vi "MicroVisco1.8.vi"() -> ()   [LabVIEW 2014]
doc: "Uses the picture indicator to display a waterfall plot. This example is similar to the Waterfall Spectrum example, which uses a multiplot graph to display a waterfall plot. However, this example can fill the area under the waveforms, because you can use the Picture VIs to fill shapes. Also, by drawing the data from back to front, this VI does not need to do the hidden line removal that the other example does.\n\nNote: You must have the LabVIEW Full or Professional Development Systems to run this example."
uses:
  Library/Image Acq..vi
  <vilib>/Utility/error.llb/DialogType.ctl
  <vilib>/Instr/_visa.llb/Select Event Type.ctl
  Library/IT_Sent.vi
  Library/SD_Sent.vi
  Library/Sent_Settings.vi
  Library/Set_OK.vi
  Library/Set_Cancel.vi
  Library/Temp_Sent.vi
  Library/Set_File_Name.vi
  Library/malfunc. stop.vi
  <vilib>/Instr/_visa.llb/VISA Configure Serial Port (Instr).vi
  <vilib>/imaqUSB/imaqUSB.llb/IMAQ USB.ctl
  <vilib>/vision/Image Controls.llb/IMAQ Image.ctl
panel:
  in  "Image File Path (jpg)":path
  out "Emer Stop ACK":string
  out "Syringe ACK":string
  out "Capture ACK":string
  out "Injection ACK":string
  out "Mode ACK":string
  out "AutoStart ACK":string
  out "Wash ACK":string
  out "Setting ACK Read":string
  out "Autostart Ind":bool=TRUE
  out "Numeric":i32
  out "Image Out (duplicate)":T1
  in  "Mal Func Stop":bool
  out "IMAQ USB Session Out 2":T2
  out "Settings ACK":bool
  out "IT Sent":dbl
  out "SD sent":dbl
  out "Sent Settings":string
  out "OK":bool
  out "Cancel":bool
  out "Temp Sent":dbl
  out "PBS Viscosity":dbl
  out "PBS Count":dbl
  out "Blood Viscosity":dbl
  out "Blood Count":dbl
  in  "Settings":bool
  out "Setting\nTemp":dbl(slide) caption="Setting \nTemperature" scale=0.0..100.0
  out "Setting \nDischarge":dbl(slide) scale=0.0..1000.0
  out "Current\nTemp":dbl(slide) caption="Current \nTemperature" scale=0.0..100.0
  out "Current \nDischarge":dbl(slide) scale=0.0..1000.0
  out "CT":dbl format="%#.1f"
  in  "Converttype":u8
  out "CD Low":string
  out "CT Low":string
  out "Stop read buffer":string
  out "Stop 2":bool
  out "CD":dbl
  out "Current RX Data":string
  out "EMER STOP ACK":bool
  out "AUTO/STRT ACK":bool
  out "MODE CTR ACK":bool
  out "SYRINGE ACK":bool
  out "CAP ACK":bool
  out "Inj ACK":bool
  out "WashACK":bool
  out "Read RX":refnum<visa-resource-name>
  in  "AutoStart":bool
  out "Syringe Ind":bool
  out "Wash Ind":bool=TRUE
  out "Inj Ind":bool
  out "Cap Ind":bool
  in  "Syringe Back":bool
  in  "capture":bool
  in  "Injection":bool
  in  "Wash":bool
  out "DATAs\nControl":i8(ring)=48 items=["STOP"=48, "Begin"=49]
  out "Commands":i8(ring)=77 items=["Torque"=84, "Fling Dist"=77, "Rotate Left"=67, "Rotate Right"=83, "Stop"=86, "Auto"=69]
  out "Checksum":i8 format="%x"
  in  "Emergency\nStop":bool
  in  "Mode Control":bool
  in  "Select COM Port":refnum<visa-resource-name>="COM1"
  out "Image Acq.":bool
  out "USB Camera Names":string[](array[string])
  out "Image out":T1
  out "IMAQ USB Session Out":T2
  out "USB Camera":string
  out "Image":T1(plugin-control)
  out "COM Port":refnum<visa-resource-name>="COM3"
  # "MICRO VISCO-METER"
  # "Auto Start"
  # "Measurements"
  # "cP"
  # "cP"
  # "o"
  # "C"
  # "uL/h"
  # "o"
  # "C"
  # "uL/h"
  # "=>"
  # "=>"
  # "=>"
  # "Syringe Release"
  # "Capture"
  # "Injection"
  # "Wash"
  # "Manual"
  # "Auto"
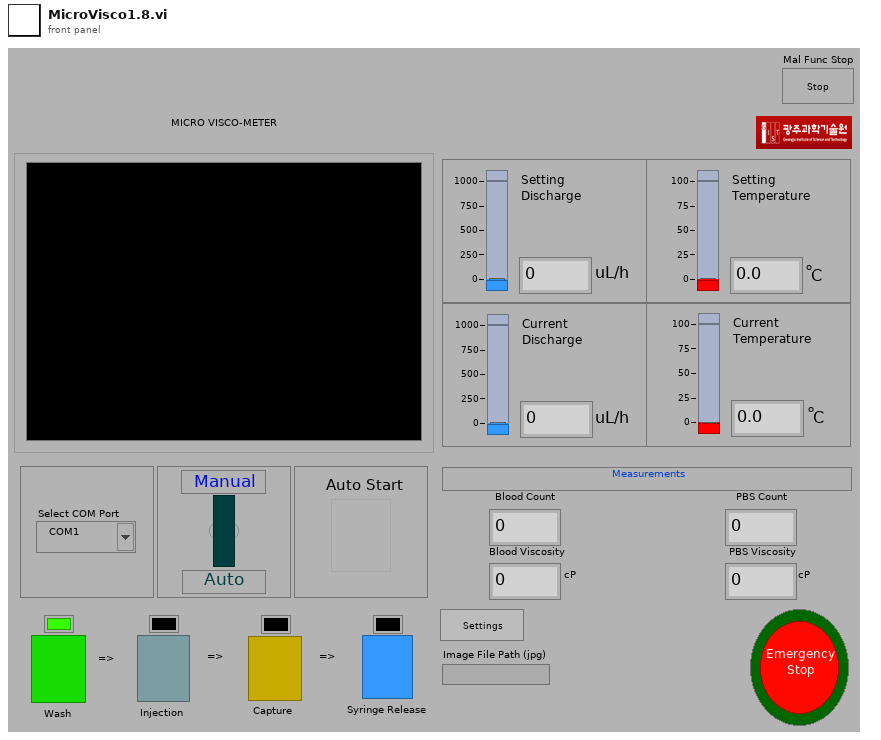
[diagram p1: front panel]
types:
  T1 = typedef "IMAQ Image.ctl" = refnum<image>
  T2 = typedef "IMAQ USB.ctl" = refnum<k1>
  T3 = enum16{"open", "replace", "create", "open or create", "replace or create", "replace or create with confirmation"}
  T4 = cluster{"xmin":dbl, "xmax":dbl, "ymin":dbl, "ymax":dbl}
  T5 = typedef "DialogType.ctl" = u16
  T6 = typedef "Select Event Type.ctl" = u32
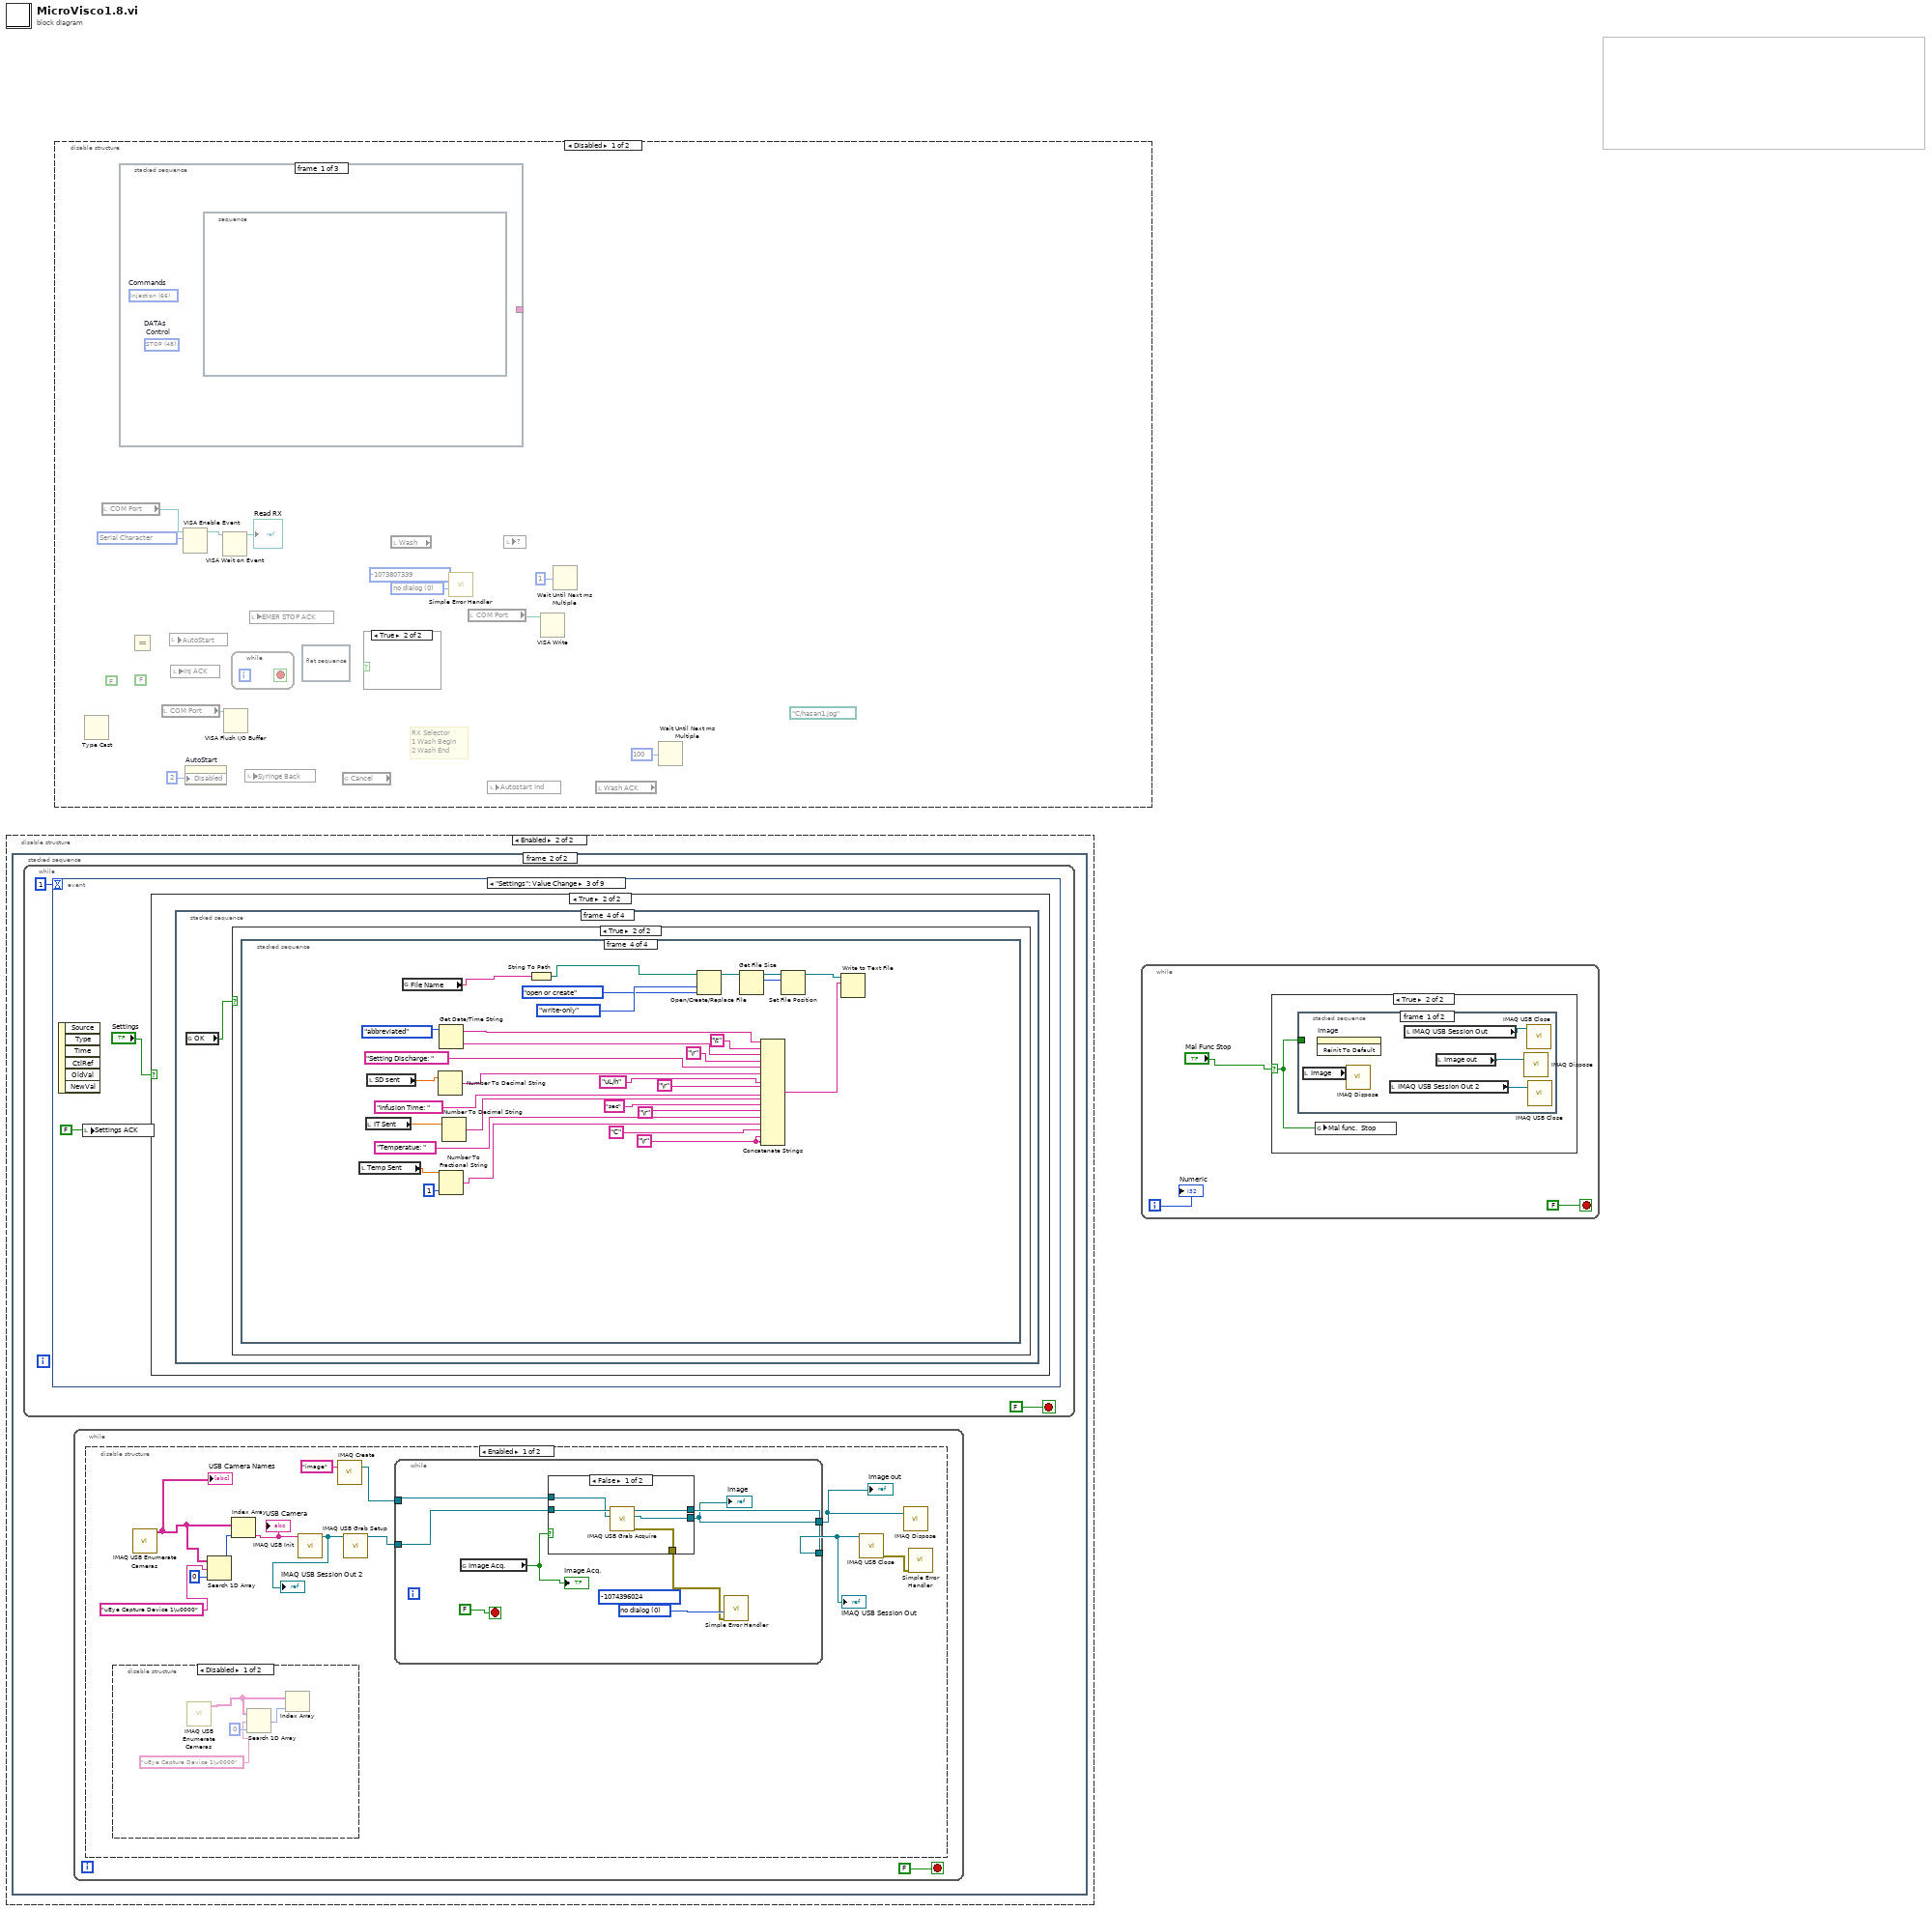
[diagram p0: block diagram]
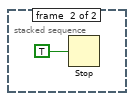
[diagram p3: hidden frame]
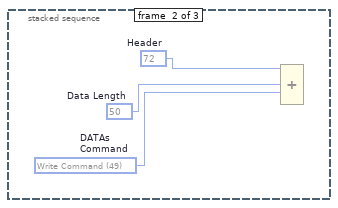
[diagram p5: hidden frame]
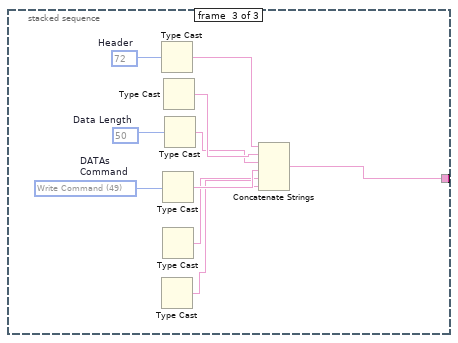
[diagram p6: hidden frame]
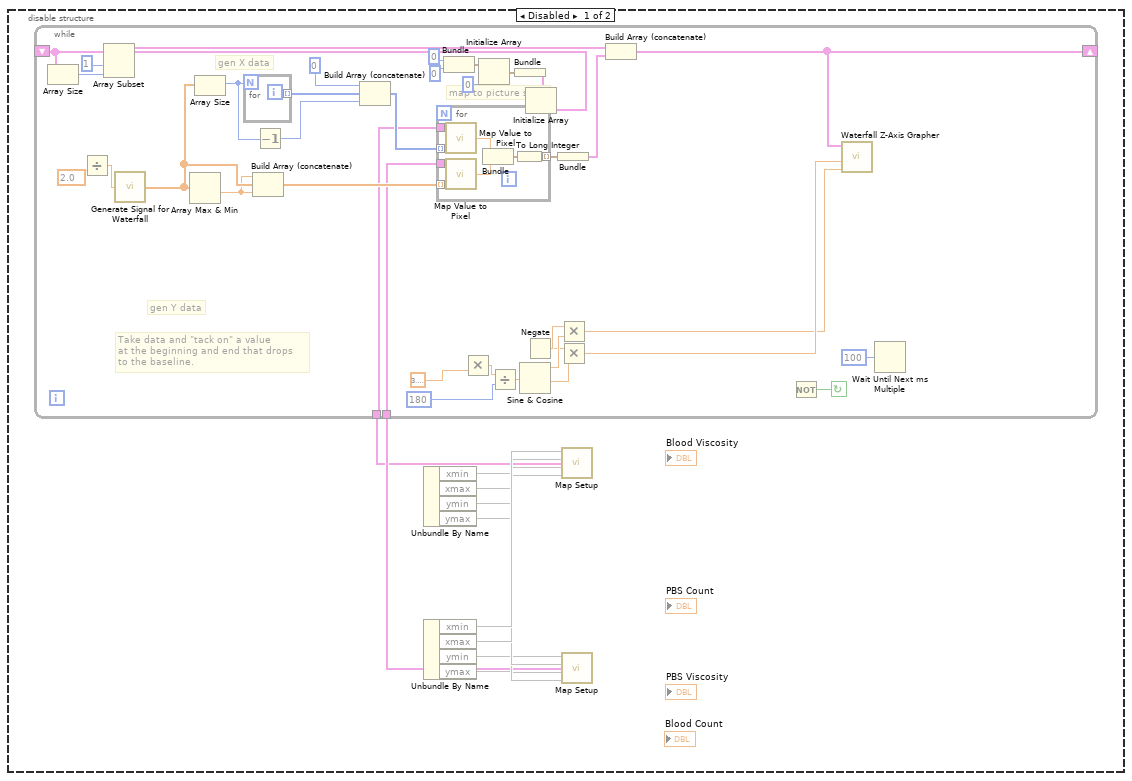
[diagram p8: hidden frame]
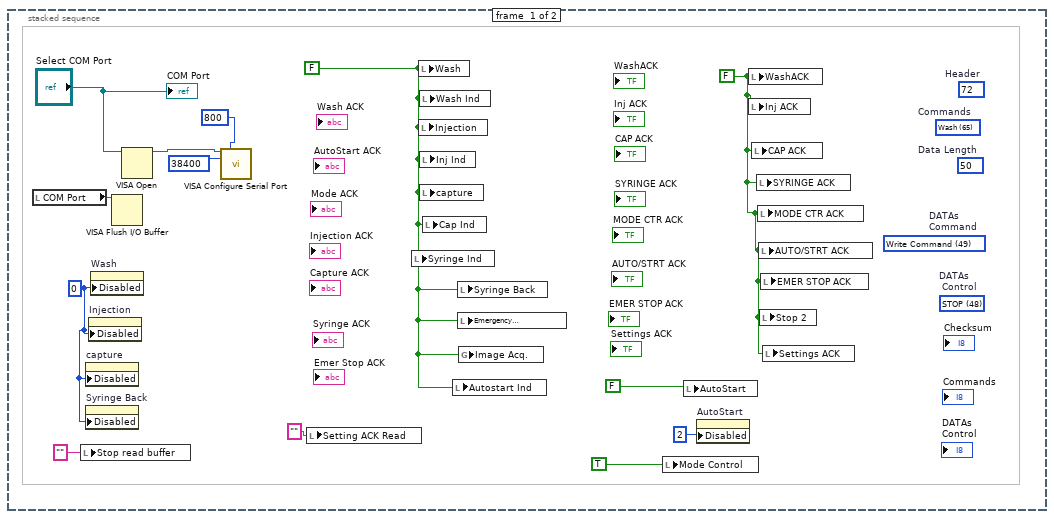
[diagram p9: hidden frame]
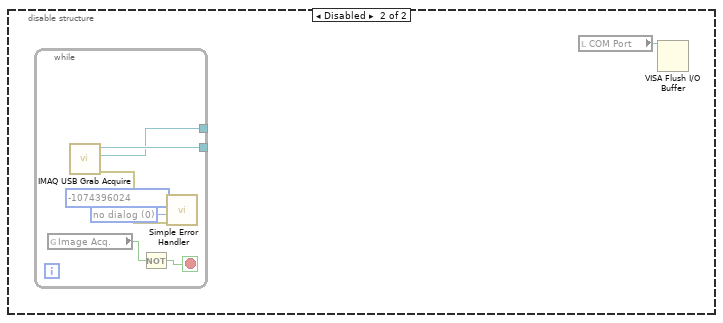
[diagram p12: hidden frame]
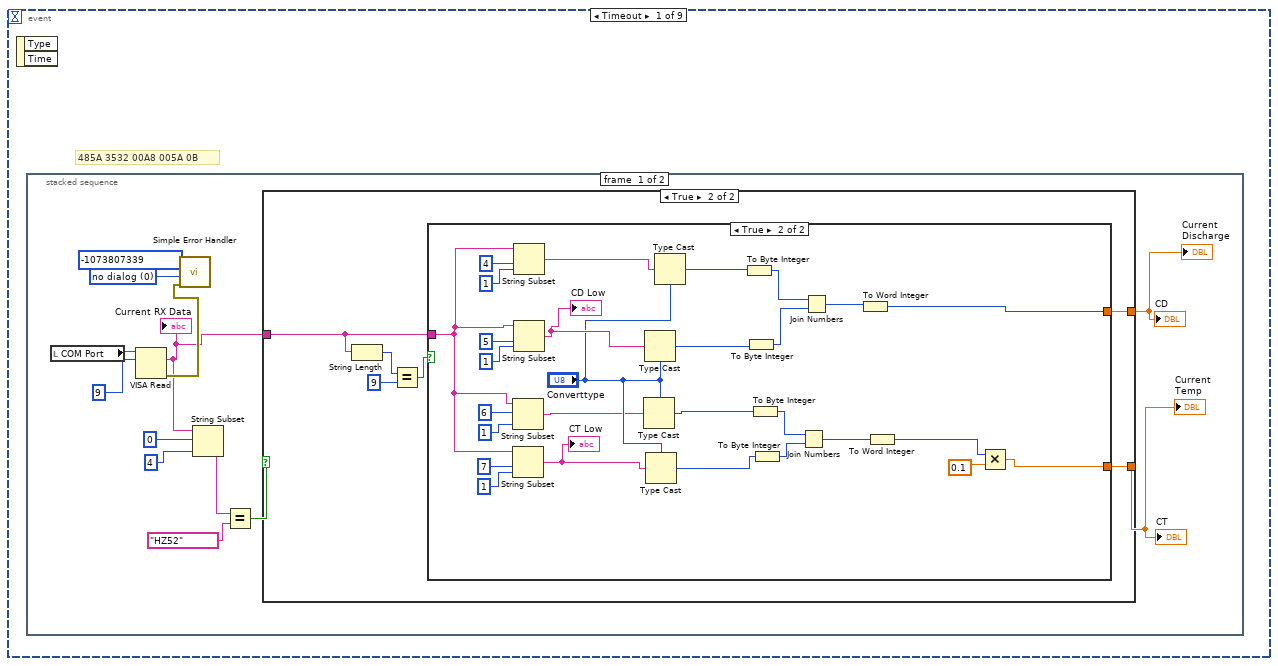
[diagram p13: hidden frame]
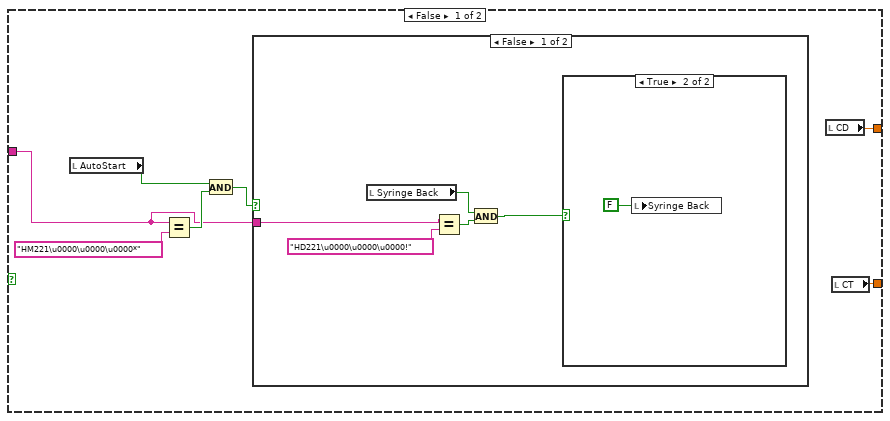
[diagram p14: hidden frame]
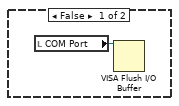
[diagram p15: hidden frame]
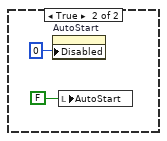
[diagram p16: hidden frame]
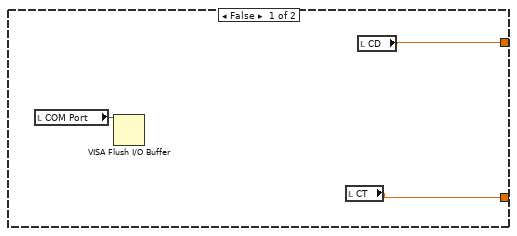
[diagram p17: hidden frame]
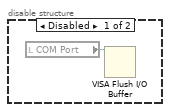
[diagram p19: hidden frame]
diagram:
  n1 = disable-structure shown="Enabled" {
    frame Disabled {
      n2 = Unbundle By Name() -> (w11:cluster{}, "xmin"=w8, "xmax"=w7, "ymin"=w6, "ymax"=w5)
      n3 = Unbundle By Name() -> (w12:T4, "xmin"=w10, "xmax"=w9, "ymin"=w4, "ymax"=w3)
      n4 = Bundle(0, 0) -> (w19:cluster{i32, i32})  [unwired: 1 in]
      n5 = Initialize Array(w19, 0) -> (w15:cluster{i32, i32}[])
      n6 = Bundle(w15) -> (w14:cluster{cluster{i32, i32}[]})  [unwired: 1 in]
      n7 = Initialize Array(w14) -> (w13:cluster{cluster{i32, i32}[]}[])  [unwired: 1 in]
      n8 = call <vilib>:"Map Setup.vi"("coordinate 1"=w10, "value 1"=w8, "coordinate 2"=w9, "value 2"=w7) -> ("scale factors"=w1:cluster{"a":dbl, "b":dbl, "log?(F)":bool})  [unwired: 1 in]
      n9 = call <vilib>:"Map Setup.vi"("coordinate 1"=w4, "value 1"=w6, "coordinate 2"=w3, "value 2"=w5) -> ("scale factors"=w2:cluster{"a":dbl, "b":dbl, "log?(F)":bool})  [unwired: 1 in]
      n10 = while {
        tunnel: w1 -> [w21]
        tunnel: w2 -> [w22]
        shift-left: w13 -> [w50]
        shift-right: [w30] -> _
        stop <- w53 continue-if-true
        # "map to picture size"
        # "Take data and \"tack on\" a value\nat the beginning and end that drops\nto the baseline."
        # "gen Y data"
        # "gen X data"
        n11 = Array Size(array=w50) -> (size(s)=w49:i32)
        n12 = Divide(y=2.0) -> (x/y=w35:dbl)  [unwired: 1 in]
        n13 = Array Subset(array=w50, index=1, length=w49) -> (w43:cluster{cluster{i32, i32}[]}[])
        n14 = call "Generate Signal for Waterfall.vi"("amplitude"=w35) -> ("waveform"=w34:dbl[], "# cycles"=w52:dbl)  [unwired: 1 in]
        n15 = Array Max & Min(array=w34) -> (min value=w33:dbl)  [unwired: 3 out]
        n16 = Array Size(array=w34) -> (size(s)=w44:i32)
        n17 = for {
          N: w44 -> [_]
          tunnel: [w63] -> w47 mode=indexing
          i -> [w63]
        }
        n18 = Build Array (concatenate)(w33, w34, w33) -> (w24:dbl[])
        n19 = Decrement(x=w44) -> (x-1=w45:i32)
        n20 = Build Array (concatenate)(0, w47, w45) -> (w25:i32[])
        n21 = for {
          tunnel: w25 -> [w62] mode=indexing
          tunnel: w24 -> [w61] mode=indexing
          tunnel: [w55] -> w23 mode=indexing
          tunnel: w22 -> [w57]
          tunnel: w21 -> [w56]
          n22 = call <vilib>:"Map Value to Pixel.vi"("x"=w62, "scale factors"=w56) -> ("pixel"=w59:dbl)  [unwired: 1 in]
          n23 = call <vilib>:"Map Value to Pixel.vi"("x"=w61, "scale factors"=w57) -> ("pixel"=w60:dbl)  [unwired: 1 in]
          n24 = Bundle("pixel"=w59, "pixel"=w60) -> (w58:cluster{"pixel":dbl, "pixel":dbl})  [unwired: 1 in]
          n25 = To Long Integer(number=w58) -> (32bit integer=w55:cluster{"pixel":i32, "pixel":i32})
        }
        n26 = Multiply(y=3.141592653589793) -> (x*y=w40:dbl)  [unwired: 1 in]
        n27 = Divide(x=w40, y=180) -> (x/y=w39:dbl)
        n28 = Sine & Cosine(0:w39) -> (1:w27:dbl, 2:w37:dbl)
        n29 = Negate() -> (x=w38:dbl, -x=w26:dbl)
        n30 = Bundle(w23) -> (w48:cluster{cluster{"pixel":i32, "pixel":i32}[]})  [unwired: 1 in]
        n31 = Multiply(x=w38, y=w27) -> (x*y=w31:dbl)
        n32 = Multiply(x=w26, y=w37) -> (x*y=w32:dbl)
        n33 = Build Array (concatenate)(w43, w48) -> (w30:cluster{cluster{"pixel":i32, "pixel":i32}[]}[])
        n34 = Not() -> (x=w54:bool, .not. x?=w53:bool)
        n35 = call "Waterfall Z-Axis Grapher.vi"("horizontal offset between plots"=w31, "vertical offset between plots"=w32, "graph"=w30) -> ("waterfall plot"=w28:picture, "colors"=w29:u32[])
        n36 = Wait Until Next ms Multiple(millisecond multiple=u32 100) -> ()  [unwired: 1 out]
      }
    }
    frame Enabled {
      n37 = stacked-sequence {
        frame #0 {
          (unwired) i8 65 items=["Syringe"=83, "Temp"=84, "Pump"=80, "Walve "=86, "LED "=76, "JIG "=74, "Wash"=65, "Injection"=66, "Capture"=67, "Readout"=68, "AUTO/MANUAL"=85, "AutoStart"=77, "E.STOP"=69, ""=0]  # Commands
          (unwired) i8 50  # Data Length
          (unwired) i8 72  # Header
          (unwired) i8 49 items=["Write Command"=49]  # DATAs Command
          (unwired) i8 48 items=["STOP"=48, "Begin"=49]  # DATAs  Control
          w70 = u8 0 ("Disabled")
          w67 = FALSE ("WashACK")
          w65 = FALSE ("Wash")
          n38 = local read "COM Port"() -> (w68:refnum<visa-resource-name>)
          n39 = local write "Stop read buffer"("" ("read buffer")) -> ()
          n40 = property on="capture" class="Bool (strict)"("Disabled"=w70) -> ()  [unwired: 2 in, 2 out]
          n41 = property on="Syringe Back" class="Bool (strict)"("Disabled"=w70) -> ()  [unwired: 2 in, 2 out]
          n42 = property on="Injection" class="Bool (strict)"("Disabled"=w70) -> ()  [unwired: 2 in, 2 out]
          n43 = property on="Wash" class="Bool (strict)"("Disabled"=w70) -> ()  [unwired: 2 in, 2 out]
          n44 = VISA Flush I/O Buffer(VISA resource name=w68) -> ()  [unwired: 1 in, 3 out]
          n45 = VISA Open(VISA resource name="Select COM Port") -> (VISA resource name=w76:refnum<visa-resource-name>)  [unwired: 1 in, 4 out]
          n46 = call-poly "VISA Configure Serial Port"("VISA resource name"=w76, "timeout (10sec)"=u32 800, "baud rate (9600)"=u32 38400) -> ()  [unwired: 4 in, 9 out]
          n47 = local write "Setting ACK Read"("" ("read buffer")) -> ()
          n48 = local write "Syringe Ind"(w65) -> ()
          n49 = local write "Wash"(w65) -> ()
          n50 = local write "Injection"(w65) -> ()
          n51 = local write "Wash Ind"(w65) -> ()
          n52 = local write "Inj Ind"(w65) -> ()
          n53 = local write "capture"(w65) -> ()
          n54 = local write "Cap Ind"(w65) -> ()
          n55 = local write "Autostart Ind"(w65) -> ()
          n56 = local write "Syringe Back"(w65) -> ()
          n57 = local write "Emergency\nStop"(w65) -> ()
          n58 = global write "Image Acq..vi" "Image Acq."(w65) -> ()
          n59 = local write "Mode Control"(TRUE ("Image Acq.")) -> ()
          n60 = local write "AutoStart"(FALSE ("AutoStart")) -> ()
          n61 = property on="AutoStart" class="Bool (strict)"("Disabled"=u8 2) -> ()  [unwired: 2 in, 2 out]
          n62 = local write "WashACK"(w67) -> ()
          n63 = local write "Inj ACK"(w67) -> ()
          n64 = local write "CAP ACK"(w67) -> ()
          n65 = local write "SYRINGE ACK"(w67) -> ()
          n66 = local write "MODE CTR ACK"(w67) -> ()
          n67 = local write "AUTO/STRT ACK"(w67) -> ()
          n68 = local write "Stop 2"(w67) -> ()
          n69 = local write "EMER STOP ACK"(w67) -> ()
          n70 = local write "Settings ACK"(w67) -> ()
          "COM Port" <- "Select COM Port"
        }
        frame #1 {
          n71 = while {
            stop <- FALSE stop-if-true
            n72 = event shown="[2] \"Settings\": Value Change" {
              selector: _ -> [_ _ _ _ _ _ _ _ _]
              dyn-events: _ -> [_ _ _ _ _ _ _ _ _]
              timeout: 1 -> [_ _ _ _ _ _ _ _ _]
              event Timeout {
                # "485A 3532 00A8 005A 0B"
                n73 = event-data() -> ()  [unwired: 3 out]
                n74 = stacked-sequence {
                  frame #0 {
                    w131 = T5 0 items=["no dialog", "OK message", "continue or stop message", "OK message + warnings", "continue/stop + warnings"] ("type of dialog (OK msg:1)")
                    n75 = local read "COM Port"() -> (w128:refnum<visa-resource-name>)
                    n76 = VISA Read(VISA resource name=w128, byte count=u32 9) -> (read buffer=w121:string, error out=w130:errorcluster)  [unwired: 1 in, 2 out]
                    "Current RX Data" <- w121
                    n77 = call <vilib>:"Simple Error Handler.vi"("error code (no error:0)"=-1073807339, "type of dialog (OK msg:1)"=w131, "error in (no error)"=w130) -> ()  [unwired: 7 out]
                    n78 = String Subset(string=w121, offset (0)=0, length (rest)=4 ("length (rest)")) -> (substring=w124:string)
                    n79 = Equal?(x=w124, y="HZ52" ("Current RX Data")) -> (x = y?=w122:bool)
                    n80 = case shown="True" w122 {
                      tunnel: w121 -> [w132 w150]
                      tunnel: [w138 w153] -> w120
                      tunnel: [w137 w152] -> w119
                      frame False {
                        n81 = local read "AutoStart"() -> (w135:bool)
                        n82 = Equal?(x=w132, y="HM221\u0000\u0000\u0000*" ("Current RX Data")) -> (x = y?=w134:bool)
                        n83 = And(x=w135, y=w134) -> (x .and. y?=w133:bool)
                        n84 = case shown="False" w133 {
                          tunnel: w132 -> [w141 _]
                          frame False {
                            n85 = local read "Syringe Back"() -> (w140:bool)
                            n86 = Equal?(x=w141, y="HD221\u0000\u0000\u0000!" ("Current RX Data")) -> (x = y?=w143:bool)
                            n87 = And(x=w140, y=w143) -> (x .and. y?=w139:bool)
                            n88 = case shown="True" w139 {
                              frame False {
                                n89 = local read "COM Port"() -> (w144:refnum<visa-resource-name>)
                                n90 = VISA Flush I/O Buffer(VISA resource name=w144) -> ()  [unwired: 1 in, 3 out]
                              }
                              frame True {
                                n91 = local write "Syringe Back"(FALSE ("Syringe Back")) -> ()
                              }
                            }
                          }
                          frame True {
                            n92 = property on="AutoStart" class="Bool (strict)"("Disabled"=u8 0) -> ()  [unwired: 2 in, 2 out]
                            n93 = local write "AutoStart"(FALSE ("AutoStart")) -> ()
                          }
                        }
                        n94 = local read "CD"() -> (w138:dbl)
                        n95 = local read "CT"() -> (w137:dbl)
                      }
                      frame True {
                        n96 = String Length(string=w150) -> (length=w149:i32)
                        n97 = Equal?(x=w149, y=9) -> (x = y?=w151:bool)
                        n98 = case shown="True" w151 {
                          tunnel: w150 -> [_ w175]
                          tunnel: [w156 w158] -> w153
                          tunnel: [w155 w157] -> w152
                          frame False {
                            n99 = local read "COM Port"() -> (w154:refnum<visa-resource-name>)
                            n100 = VISA Flush I/O Buffer(VISA resource name=w154) -> ()  [unwired: 1 in, 3 out]
                            n101 = local read "CT"() -> (w155:dbl)
                            n102 = local read "CD"() -> (w156:dbl)
                          }
                          frame True {
                            n103 = String Subset(string=w175, offset (0)=6, length (rest)=1 ("length (rest)")) -> (substring=w164:string)
                            n104 = String Subset(string=w175, offset (0)=7, length (rest)=1 ("length (rest)")) -> (substring=w161:string)
                            "CT Low" <- w161
                            n105 = String Subset(string=w175, offset (0)=4, length (rest)=1 ("length (rest)")) -> (substring=w167:string)
                            n106 = String Subset(string=w175, offset (0)=5, length (rest)=1 ("length (rest)")) -> (substring=w166:string)
                            "CD Low" <- w166
                            n107 = Type Cast(type="Converttype", x=w164) -> (*(type *) &x=w163:u8)
                            n108 = Type Cast(type="Converttype", x=w166) -> (*(type *) &x=w168:u8)
                            n109 = Type Cast(type="Converttype", x=w161) -> (*(type *) &x=w162:u8)
                            n110 = Type Cast(type="Converttype", x=w167) -> (*(type *) &x=w169:u8)
                            n111 = To Byte Integer(number=w169) -> (8bit integer=w171:i8)
                            n112 = To Byte Integer(number=w168) -> (8bit integer=w170:i8)
                            n113 = To Byte Integer(number=w163) -> (8bit integer=w174:i8)
                            n114 = To Byte Integer(number=w162) -> (8bit integer=w160:i8)
                            n115 = Join Numbers(hi=w174, lo=w160) -> ((hi.lo)=w159:u16)
                            n116 = Join Numbers(hi=w171, lo=w170) -> ((hi.lo)=w176:u16)
                            n117 = To Word Integer(number=w176) -> (16bit integer=w158:i16)
                            n118 = To Word Integer(number=w159) -> (16bit integer=w172:i16)
                            n119 = Multiply(x=w172, y=0.1 ("Numeric")) -> (x*y=w157:dbl)
                          }
                        }
                      }
                    }
                    "CD" <- w120
                    "CT" <- w119
                    "Current \nDischarge" <- w120
                    "Current\nTemp" <- w119
                  }
                  frame #1 {
                    n120 = disable-structure shown="Enabled" {
                      frame Enabled {
                        # "Only for Test"
                      }
                      frame Disabled {
                      }
                    }
                    n121 = disable-structure shown="Enabled" {
                      frame Disabled {
                        n122 = local read "COM Port"() -> (w185:refnum<visa-resource-name>)
                        n123 = VISA Flush I/O Buffer(VISA resource name=w185) -> ()  [unwired: 1 in, 3 out]
                      }
                      frame Enabled {
                      }
                    }
                  }
                }
              }
              event "Mode Control": Value Change {
                w187 = i8 85 items=["Syringe"=83, "Temp"=84, "Pump"=80, "Walve "=86, "LED "=76, "JIG "=74, "Wash"=65, "Injection"=66, "Capture"=67, "Readout"=68, "AUTO/MANUAL"=85, "E.STOP"=69]  # Commands
                n124 = event-data() -> ()  [unwired: 7 out]
                n125 = local write "Commands"(w187) -> ()
                n126 = local write "MODE CTR ACK"(FALSE ("MODE CTR ACK")) -> ()
                n127 = case shown="True" "Mode Control" {
                  frame False {
                    w189 = FALSE ("Wash")
                    n128 = local write "Wash Ind"(w189) -> ()
                    n129 = local write "Injection"(w189) -> ()
                    n130 = local write "Wash"(w189) -> ()
                    n131 = local write "Inj Ind"(w189) -> ()
                    n132 = local write "capture"(w189) -> ()
                    n133 = local write "Cap Ind"(w189) -> ()
                    n134 = local write "Syringe Back"(w189) -> ()
                    n135 = local write "Syringe Ind"(w189) -> ()
                    n136 = stacked-sequence {
                      frame #0 {
                        n137 = local read "COM Port"() -> (w190:refnum<visa-resource-name>)
                        n138 = VISA Flush I/O Buffer(VISA resource name=w190) -> ()  [unwired: 1 in, 3 out]
                      }
                      frame #1 {
                        w191 = i8 49 items=["MANUAL"=50, "AUTO"=49]  # DATAs  Control
                        n139 = local write "DATAs\nControl"(w191) -> ()
                      }
                      frame #2 {
                        w194 = i8 49 items=["Write Command"=49]  # DATAs Command
                        w196 = i8 50  # Data Length
                        w197 = i8 72  # Header
                        n140 = local read "Commands"() -> (w195:i8)
                        n141 = local read "DATAs\nControl"() -> (w193:i8)
                        n142 = Compound Arithmetic op=ADD(w197, w195, w196, w194, w193) -> (w192:i8)
                        n143 = local write "Checksum"(w192) -> ()
                      }
                      frame #3 {
                        n144 = flat-sequence {
                          frame #0 {
                            w210 = i8 50  # Data Length
                            w211 = i8 72  # Header
                            w209 = i8 49 items=["Write Command"=49]  # DATAs Command
                            n145 = local read "DATAs\nControl"() -> (w201:i8)
                            n146 = local read "Checksum"() -> (w200:i8)
                            n147 = local read "Commands"() -> (w202:i8)
                            n148 = Type Cast(x=w211) -> (*(type *) &x=w208:string)  [unwired: 1 out]
                            n149 = Type Cast(x=w200) -> (*(type *) &x=w203:string)  [unwired: 1 out]
                            n150 = Type Cast(x=w209) -> (*(type *) &x=w205:string)  [unwired: 1 out]
                            n151 = Type Cast(x=w201) -> (*(type *) &x=w204:string)  [unwired: 1 out]
                            n152 = Type Cast(x=w202) -> (*(type *) &x=w207:string)  [unwired: 1 out]
                            n153 = Type Cast(x=w210) -> (*(type *) &x=w206:string)  [unwired: 1 out]
                            n154 = Concatenate Strings(w208, w207, w206, w205, w204, w203) -> (w198:string)
                            n155 = local read "COM Port"() -> (w199:refnum<visa-resource-name>)
                            n156 = VISA Write(VISA resource name=w199, write buffer=w198) -> ()  [unwired: 1 in, 3 out]
                          }
                          frame #1 {
                            n157 = local read "COM Port"() -> (w212:refnum<visa-resource-name>)
                            n158 = VISA Read(VISA resource name=w212, byte count=u32 6) -> (read buffer=w214:string)  [unwired: 1 in, 3 out]
                            n159 = local write "Mode ACK"(w214) -> ()
                          }
                        }
                      }
                      frame #4 {
                        n160 = while {
                          stop <- w215 stop-if-true
                          n161 = flat-sequence {
                            frame #0 {
                              w220 = "HU\u0015\u0000\u0000²"  # Auto Ctrl NACK
                              w218 = "HU2111"  # Auto Control
                              n162 = local read "Mode ACK"() -> (w217:string)
                              n163 = local read "COM Port"() -> (w216:refnum<visa-resource-name>)
                              n164 = Equal?(x=w217, y=w218) -> (x = y?=w221:bool)
                              n165 = Equal?(x=w217, y=w220) -> (x = y?=w219:bool)
                              n166 = case shown="True" w221 {
                                tunnel: w219 -> [w224 _]
                                tunnel: w216 -> [w223 _]
                                tunnel: w218 -> [w222 _]
                                frame False {
                                n167 = case shown="True" w224 {
                                tunnel: w223 -> [w226 w229]
                                tunnel: w222 -> [w225 w228]
                                frame False {
                                n168 = local write "MODE CTR ACK"(FALSE ("MODE CTR ACK")) -> ()
                                n169 = VISA Write(VISA resource name=w226, write buffer=w225) -> ()  [unwired: 1 in, 3 out]
                                }
                                frame True {
                                n170 = local write "MODE CTR ACK"(FALSE ("MODE CTR ACK")) -> ()
                                n171 = VISA Write(VISA resource name=w229, write buffer=w228) -> ()  [unwired: 1 in, 3 out]
                                }
                                }
                                }
                                frame True {
                                w232 = u8 2 ("Disabled")
                                n172 = property on="Injection" class="Bool (strict)"("Disabled"=w232) -> ()  [unwired: 2 in, 2 out]
                                n173 = property on="Wash" class="Bool (strict)"("Disabled"=w232) -> ()  [unwired: 2 in, 2 out]
                                n174 = local write "MODE CTR ACK"(TRUE ("MODE CTR ACK")) -> ()
                                n175 = property on="capture" class="Bool (strict)"("Disabled"=w232) -> ()  [unwired: 2 in, 2 out]
                                n176 = property on="Syringe Back" class="Bool (strict)"("Disabled"=w232) -> ()  [unwired: 2 in, 2 out]
                                n177 = property on="AutoStart" class="Bool (strict)"("Disabled"=u8 0) -> ()  [unwired: 2 in, 2 out]
                                }
                              }
                            }
                            frame #1 {
                              n178 = local read "COM Port"() -> (w234:refnum<visa-resource-name>)
                              n179 = VISA Flush I/O Buffer(VISA resource name=w234) -> ()  [unwired: 1 in, 3 out]
                            }
                          }
                          n180 = local read "MODE CTR ACK"() -> (w215:bool)
                        }
                      }
                    }
                  }
                  frame True {
                    n181 = stacked-sequence {
                      frame #0 {
                        n182 = local read "COM Port"() -> (w235:refnum<visa-resource-name>)
                        n183 = VISA Flush I/O Buffer(VISA resource name=w235) -> ()  [unwired: 1 in, 3 out]
                      }
                      frame #1 {
                        w236 = i8 50 items=["MANUAL"=50, "AUTO"=49]  # DATAs  Control
                        n184 = local write "DATAs\nControl"(w236) -> ()
                      }
                      frame #2 {
                        w239 = i8 49 items=["Write Command"=49]  # DATAs Command
                        w241 = i8 50  # Data Length
                        w242 = i8 72  # Header
                        n185 = local read "DATAs\nControl"() -> (w238:i8)
                        n186 = local read "Commands"() -> (w240:i8)
                        n187 = Compound Arithmetic op=ADD(w242, w240, w241, w239, w238) -> (w237:i8)
                        n188 = local write "Checksum"(w237) -> ()
                      }
                      frame #3 {
                        n189 = flat-sequence {
                          frame #0 {
                            w255 = i8 50  # Data Length
                            w256 = i8 72  # Header
                            w254 = i8 49 items=["Write Command"=49]  # DATAs Command
                            n190 = local read "DATAs\nControl"() -> (w246:i8)
                            n191 = local read "Commands"() -> (w247:i8)
                            n192 = local read "Checksum"() -> (w245:i8)
                            n193 = Type Cast(x=w256) -> (*(type *) &x=w253:string)  [unwired: 1 out]
                            n194 = Type Cast(x=w245) -> (*(type *) &x=w248:string)  [unwired: 1 out]
                            n195 = Type Cast(x=w254) -> (*(type *) &x=w250:string)  [unwired: 1 out]
                            n196 = Type Cast(x=w246) -> (*(type *) &x=w249:string)  [unwired: 1 out]
                            n197 = Type Cast(x=w247) -> (*(type *) &x=w252:string)  [unwired: 1 out]
                            n198 = Type Cast(x=w255) -> (*(type *) &x=w251:string)  [unwired: 1 out]
                            n199 = Concatenate Strings(w253, w252, w251, w250, w249, w248) -> (w243:string)
                            n200 = local read "COM Port"() -> (w244:refnum<visa-resource-name>)
                            n201 = VISA Write(VISA resource name=w244, write buffer=w243) -> ()  [unwired: 1 in, 3 out]
                          }
                          frame #1 {
                            n202 = local read "COM Port"() -> (w259:refnum<visa-resource-name>)
                            n203 = VISA Read(VISA resource name=w259, byte count=u32 6) -> (read buffer=w257:string)  [unwired: 1 in, 3 out]
                            n204 = local write "Mode ACK"(w257) -> ()
                          }
                        }
                      }
                      frame #4 {
                        n205 = while {
                          stop <- w260 stop-if-true
                          n206 = flat-sequence {
                            frame #0 {
                              w261 = "HU2122"  # Manual Ctrl
                              w265 = "HU\u0015\u0000\u0000²"  # Auto Ctrl NACK
                              n207 = local read "Mode ACK"() -> (w263:string)
                              n208 = local read "COM Port"() -> (w262:refnum<visa-resource-name>)
                              n209 = Equal?(x=w263, y=w261) -> (x = y?=w266:bool)
                              n210 = Equal?(x=w263, y=w265) -> (x = y?=w264:bool)
                              n211 = case shown="True" w266 {
                                tunnel: w264 -> [w269 _]
                                tunnel: w262 -> [w268 _]
                                tunnel: w261 -> [w267 _]
                                frame False {
                                n212 = case shown="True" w269 {
                                tunnel: w268 -> [w271 w274]
                                tunnel: w267 -> [w270 w273]
                                frame False {
                                n213 = local write "MODE CTR ACK"(FALSE ("MODE CTR ACK")) -> ()
                                n214 = VISA Write(VISA resource name=w271, write buffer=w270) -> ()  [unwired: 1 in, 3 out]
                                }
                                frame True {
                                n215 = local write "MODE CTR ACK"(FALSE ("MODE CTR ACK")) -> ()
                                n216 = VISA Write(VISA resource name=w274, write buffer=w273) -> ()  [unwired: 1 in, 3 out]
                                }
                                }
                                }
                                frame True {
                                w277 = u8 0 ("Disabled")
                                n217 = property on="Injection" class="Bool (strict)"("Disabled"=w277) -> ()  [unwired: 2 in, 2 out]
                                n218 = property on="Wash" class="Bool (strict)"("Disabled"=w277) -> ()  [unwired: 2 in, 2 out]
                                n219 = local write "MODE CTR ACK"(TRUE ("MODE CTR ACK")) -> ()
                                n220 = property on="capture" class="Bool (strict)"("Disabled"=w277) -> ()  [unwired: 2 in, 2 out]
                                n221 = property on="Syringe Back" class="Bool (strict)"("Disabled"=w277) -> ()  [unwired: 2 in, 2 out]
                                n222 = property on="AutoStart" class="Bool (strict)"("Disabled"=u8 2) -> ()  [unwired: 2 in, 2 out]
                                }
                              }
                            }
                            frame #1 {
                              n223 = local read "COM Port"() -> (w279:refnum<visa-resource-name>)
                              n224 = VISA Flush I/O Buffer(VISA resource name=w279) -> ()  [unwired: 1 in, 3 out]
                            }
                          }
                          n225 = local read "MODE CTR ACK"() -> (w260:bool)
                        }
                      }
                    }
                  }
                }
              }
              event "Settings": Value Change {
                n226 = event-data() -> ()  [unwired: 7 out]
                n227 = local write "Settings ACK"(FALSE ("Settings ACK")) -> ()
                n228 = case shown="True" "Settings" {
                  frame False {
                  }
                  frame True {
                    n229 = stacked-sequence {
                      frame #0 {
                        n230 = local read "COM Port"() -> (w282:refnum<visa-resource-name>)
                        n231 = VISA Flush I/O Buffer(VISA resource name=w282) -> ()  [unwired: 1 in, 3 out]
                      }
                      frame #1 {
                        n232 = call "Settings1.1.vi"() -> ()  [unwired: 1 out]
                      }
                      frame #2 {
                        n233 = global read "Sent_Settings.vi" "Sent Settings"() -> (→"Sent Settings":string)
                        n234 = global read "Temp_Sent.vi" "Temp Sent"() -> (→"Temp Sent" →"Setting\nTemp":dbl)
                        n235 = global read "IT_Sent.vi" "IT Sent"() -> (→"IT Sent":dbl)
                        n236 = global read "SD_Sent.vi" "SD sent"() -> (→"SD sent" →"Setting \nDischarge":dbl)
                        n237 = global read "Set_Cancel.vi" "Cancel"() -> (→"Cancel":bool)
                        n238 = global read "Set_OK.vi" "OK"() -> (→"OK":bool)
                      }
                      frame #3 {
                        n239 = global read "Set_OK.vi" "OK"() -> (w289:bool)
                        n240 = case shown="True" w289 {
                          frame False {
                          }
                          frame True {
                            n241 = stacked-sequence {
                              frame #0 {
                                n242 = local read "COM Port"() -> (w291:refnum<visa-resource-name>)
                                n243 = VISA Flush I/O Buffer(VISA resource name=w291) -> ()  [unwired: 1 in, 3 out]
                                n244 = Wait Until Next ms Multiple(millisecond multiple=u32 1) -> ()  [unwired: 1 out]
                              }
                              frame #1 {
                                n245 = flat-sequence {
                                tunnel: [w298] -> w293
                                tunnel: [w301] -> w294
                                frame #0 {
                                n246 = global read "Sent_Settings.vi" "Sent Settings"() -> (w296:string)
                                n247 = local read "COM Port"() -> (w295:refnum<visa-resource-name>)
                                n248 = VISA Write(VISA resource name=w295, write buffer=w296) -> ()  [unwired: 1 in, 3 out]
                                }
                                frame #1 {
                                n249 = Wait Until Next ms Multiple(millisecond multiple=u32 1) -> ()  [unwired: 1 out]
                                }
                                frame #2 {
                                n250 = local read "COM Port"() -> (w299:refnum<visa-resource-name>)
                                n251 = VISA Read(VISA resource name=w299, byte count=u32 8) -> (read buffer=w298:string)  [unwired: 1 in, 3 out]
                                }
                                frame #3 {
                                n252 = local read "COM Port"() -> (w303:refnum<visa-resource-name>)
                                n253 = VISA Read(VISA resource name=w303, byte count=u32 3) -> (read buffer=w301:string)  [unwired: 1 in, 3 out]
                                }
                                }
                                n254 = Concatenate Strings(w293, w294) -> (→"Setting ACK Read":string)
                              }
                              frame #2 {
                                (unwired) 20
                                n255 = while {
                                stop <- w304 stop-if-true
                                n256 = flat-sequence {
                                frame #0 {
                                w309 = "HY\u0015\u0000\u0000\u0000\u0000\u0000\u0000\u0000¶"  # Auto Ctrl NACK
                                n257 = local read "Setting ACK Read"() -> (w305:string)
                                n258 = local read "Sent Settings"() -> (w306:string)
                                n259 = Equal?(x=w305, y=w306) -> (x = y?=w308:bool)
                                n260 = Equal?(x=w305, y=w309) -> (x = y?=w307:bool)
                                n261 = case shown="False" w308 {
                                tunnel: w307 -> [w311 _]
                                tunnel: w306 -> [w310 _]
                                frame False {
                                n262 = case shown="False" w311 {
                                tunnel: w310 -> [w312 w317]
                                frame False {
                                n263 = stacked-sequence {
                                tunnel: w312 -> [_ w315]
                                frame #0 {
                                n264 = local read "COM Port"() -> (w313:refnum<visa-resource-name>)
                                n265 = VISA Flush I/O Buffer(VISA resource name=w313) -> ()  [unwired: 1 in, 3 out]
                                }
                                frame #1 {
                                n266 = local read "COM Port"() -> (w316:refnum<visa-resource-name>)
                                n267 = local write "Settings ACK"(FALSE ("Settings ACK")) -> ()
                                n268 = VISA Write(VISA resource name=w316, write buffer=w315) -> ()  [unwired: 1 in, 3 out]
                                }
                                }
                                }
                                frame True {
                                n269 = stacked-sequence {
                                tunnel: w317 -> [_ w320]
                                frame #0 {
                                n270 = local read "COM Port"() -> (w318:refnum<visa-resource-name>)
                                n271 = VISA Flush I/O Buffer(VISA resource name=w318) -> ()  [unwired: 1 in, 3 out]
                                }
                                frame #1 {
                                n272 = local read "COM Port"() -> (w321:refnum<visa-resource-name>)
                                n273 = local write "Settings ACK"(FALSE ("Settings ACK")) -> ()
                                n274 = VISA Write(VISA resource name=w321, write buffer=w320) -> ()  [unwired: 1 in, 3 out]
                                }
                                }
                                }
                                }
                                }
                                frame True {
                                n275 = local write "Settings ACK"(TRUE ("Settings ACK")) -> ()
                                }
                                }
                                }
                                }
                                n276 = local read "Settings ACK"() -> (w304:bool)
                                }
                              }
                              frame #3 {
                                w327 = "\r"
                                n277 = local read "Temp Sent"() -> (w325:dbl)
                                n278 = local read "IT Sent"() -> (w342:dbl)
                                n279 = local read "SD sent"() -> (w347:dbl)
                                n280 = global read "Set_File_Name.vi" "File Name"() -> (w323:string)
                                n281 = Number To Decimal String(number=w347) -> (decimal integer string=w346:string)  [unwired: 1 out]
                                n282 = Get Date/Time String(date format (0)=enum16{"short", "long", "abbreviated"}."abbreviated") -> (date string=w351:string, time string=w350:string)  [unwired: 2 out]
                                n283 = Number To Fractional String(number=w325, precision (6)=i16 1) -> (F-format string=w324:string)  [unwired: 2 out]
                                n284 = Number To Decimal String(number=w342) -> (decimal integer string=w341:string)  [unwired: 1 out]
                                n285 = String To Path(string=w323) -> (path=w333:path)
                                n286 = Open/Create/Replace File(file path (use dialog)=w333, operation (0:open)=T3."open or create", access (0:read/write)=enum16{"read/write", "read-only", "write-only"}."write-only") -> (refnum out=w332:refnum<file>)  [unwired: 1 in, 4 out]
                                n287 = Get File Size(file=w332) -> (refnum out=w335:refnum<file>, size (in bytes)=w336:i64)  [unwired: 1 in, 1 out]
                                n288 = Concatenate Strings(w351, "\t", w350, "\r", "Setting Discharge: ", w346, "uL/h" ("string"), "\r", "Infusion Time: ", w341, "sec" ("string"), "\r", "Temperatue: ", w324, "C" ("string"), w327, w327) -> (w331:string)
                                n289 = Set File Position(offset (in bytes) (0)=w336, refnum=w335) -> (refnum out=w334:refnum<file>)  [unwired: 1 in, 2 out]
                                n290 = Write to Text File(file (use dialog)=w334, text=w331) -> ()  [unwired: 1 in, 4 out]
                              }
                            }
                          }
                        }
                      }
                    }
                  }
                }
              }
              event "AutoStart": Value Change {
                w354 = i8 77 items=["Syringe"=83, "Temp"=84, "Pump"=80, "Walve "=86, "LED "=76, "JIG "=74, "Wash"=65, "Injection"=66, "Capture"=67, "Readout"=68, "AUTO/MANUAL"=85, "AutoStart"=77, "E.STOP"=69]  # Commands
                n291 = event-data() -> ()  [unwired: 7 out]
                n292 = local write "Commands"(w354) -> ()
                n293 = local write "AUTO/STRT ACK"(FALSE ("AUTO/STRT ACK")) -> ()
                n294 = disable-structure shown="Enabled" {
                  disable-tunnel: "AutoStart" -> [w356 _]
                  frame Enabled {
                    n295 = case shown="True" w356 {
                      selector: w356 -> [w357 w405]
                      frame False {
                        n296 = local write "Autostart Ind"(w357) -> ()
                        n297 = disable-structure shown="Disabled" {
                          frame Disabled {
                            n298 = stacked-sequence {
                              frame #0 {
                                n299 = local read "COM Port"() -> (w358:refnum<visa-resource-name>)
                                n300 = VISA Flush I/O Buffer(VISA resource name=w358) -> ()  [unwired: 1 in, 3 out]
                              }
                              frame #1 {
                                w359 = i8 48 items=["MANUAL"=48, "AUTO"=49]  # DATAs  Control
                                n301 = local write "DATAs\nControl"(w359) -> ()
                              }
                              frame #2 {
                                w362 = i8 49 items=["Write Command"=49]  # DATAs Command
                                w361 = i8 50  # Data Length
                                w360 = i8 72  # Header
                                n302 = local read "Commands"() -> (w363:i8)
                                n303 = local read "DATAs\nControl"() -> (w364:i8)
                                n304 = Compound Arithmetic op=ADD(w360, w363, w361, w362, w364) -> (w365:i8)
                                n305 = local write "Checksum"(w365) -> ()
                              }
                              frame #3 {
                                w378 = i8 50  # Data Length
                                w379 = i8 72  # Header
                                w377 = i8 49 items=["Write Command"=49]  # DATAs Command
                                n306 = local read "Commands"() -> (w368:i8)
                                n307 = local read "DATAs\nControl"() -> (w367:i8)
                                n308 = local read "Checksum"() -> (w366:i8)
                                n309 = Type Cast(x=w379) -> (*(type *) &x=w376:string)  [unwired: 1 out]
                                n310 = Type Cast(x=w366) -> (*(type *) &x=w371:string)  [unwired: 1 out]
                                n311 = Type Cast(x=w377) -> (*(type *) &x=w373:string)  [unwired: 1 out]
                                n312 = Type Cast(x=w367) -> (*(type *) &x=w372:string)  [unwired: 1 out]
                                n313 = Type Cast(x=w368) -> (*(type *) &x=w375:string)  [unwired: 1 out]
                                n314 = Type Cast(x=w378) -> (*(type *) &x=w374:string)  [unwired: 1 out]
                                n315 = Concatenate Strings(w376, w375, w374, w373, w372, w371) -> (w369:string)
                                n316 = local read "COM Port"() -> (w370:refnum<visa-resource-name>)
                                n317 = VISA Write(VISA resource name=w370, write buffer=w369) -> ()  [unwired: 1 in, 3 out]
                              }
                              frame #4 {
                                n318 = while {
                                stop <- w382 stop-if-true
                                n319 = flat-sequence {
                                tunnel: [w385] -> w383
                                tunnel: [w385] -> w381
                                tunnel: [w384] -> w380
                                tunnel: w383 -> [w393]
                                tunnel: w381 -> [w390]
                                tunnel: w380 -> [w388]
                                frame #0 {
                                n320 = local read "COM Port"() -> (w384:refnum<visa-resource-name>)
                                n321 = VISA Read(VISA resource name=w384, byte count=u32 6) -> (read buffer=w385:string)  [unwired: 1 in, 3 out]
                                }
                                frame #1 {
                                w387 = "HM210("  # AutoStop
                                w391 = "HM\u0015\u0000\u0000ª"  # AutoStart NACK
                                n322 = Equal?(x=w393, y=w387) -> (x = y?=w392:bool)
                                n323 = Equal?(x=w390, y=w391) -> (x = y?=w389:bool)
                                n324 = case shown="False" w392 {
                                tunnel: w389 -> [w396 _]
                                tunnel: w388 -> [w395 _]
                                tunnel: w387 -> [w394 _]
                                frame False {
                                n325 = case shown="False" w396 {
                                tunnel: w395 -> [w398 w401]
                                tunnel: w394 -> [w397 w400]
                                frame False {
                                n326 = local write "AUTO/STRT ACK"(FALSE ("AUTO/STRT ACK")) -> ()
                                n327 = VISA Write(VISA resource name=w398, write buffer=w397) -> ()  [unwired: 1 in, 3 out]
                                }
                                frame True {
                                n328 = local write "AUTO/STRT ACK"(FALSE ("AUTO/STRT ACK")) -> ()
                                n329 = VISA Write(VISA resource name=w401, write buffer=w400) -> ()  [unwired: 1 in, 3 out]
                                }
                                }
                                }
                                frame True {
                                n330 = local write "AUTO/STRT ACK"(TRUE ("AUTO/STRT ACK")) -> ()
                                }
                                }
                                }
                                frame #2 {
                                n331 = local read "COM Port"() -> (w404:refnum<visa-resource-name>)
                                n332 = VISA Flush I/O Buffer(VISA resource name=w404) -> ()  [unwired: 1 in, 3 out]
                                }
                                }
                                n333 = local read "AUTO/STRT ACK"() -> (w382:bool)
                                }
                              }
                            }
                          }
                          frame Enabled {
                          }
                        }
                      }
                      frame True {
                        n334 = stacked-sequence {
                          frame #0 {
                            n335 = local read "COM Port"() -> (w406:refnum<visa-resource-name>)
                            n336 = VISA Flush I/O Buffer(VISA resource name=w406) -> ()  [unwired: 1 in, 3 out]
                          }
                          frame #1 {
                            w407 = i8 49 items=["MANUAL"=48, "AUTO"=49]  # DATAs  Control
                            n337 = local write "DATAs\nControl"(w407) -> ()
                          }
                          frame #2 {
                            w411 = i8 49 items=["Write Command"=49]  # DATAs Command
                            w412 = i8 50  # Data Length
                            w413 = i8 72  # Header
                            n338 = local read "Commands"() -> (w410:i8)
                            n339 = local read "DATAs\nControl"() -> (w409:i8)
                            n340 = Compound Arithmetic op=ADD(w413, w410, w412, w411, w409) -> (w408:i8)
                            n341 = local write "Checksum"(w408) -> ()
                          }
                          frame #3 {
                            n342 = flat-sequence {
                              frame #0 {
                                w427 = i8 50  # Data Length
                                w419 = i8 72  # Header
                                w426 = i8 49 items=["Write Command"=49]  # DATAs Command
                                n343 = local read "Commands"() -> (w418:i8)
                                n344 = local read "DATAs\nControl"() -> (w416:i8)
                                n345 = local read "Checksum"() -> (w417:i8)
                                n346 = Type Cast(x=w419) -> (*(type *) &x=w425:string)  [unwired: 1 out]
                                n347 = Type Cast(x=w417) -> (*(type *) &x=w420:string)  [unwired: 1 out]
                                n348 = Type Cast(x=w426) -> (*(type *) &x=w422:string)  [unwired: 1 out]
                                n349 = Type Cast(x=w416) -> (*(type *) &x=w421:string)  [unwired: 1 out]
                                n350 = Type Cast(x=w418) -> (*(type *) &x=w424:string)  [unwired: 1 out]
                                n351 = Type Cast(x=w427) -> (*(type *) &x=w423:string)  [unwired: 1 out]
                                n352 = Concatenate Strings(w425, w424, w423, w422, w421, w420) -> (w414:string)
                                n353 = local read "COM Port"() -> (w415:refnum<visa-resource-name>)
                                n354 = VISA Write(VISA resource name=w415, write buffer=w414) -> ()  [unwired: 1 in, 3 out]
                              }
                              frame #1 {
                                n355 = local read "COM Port"() -> (w429:refnum<visa-resource-name>)
                                n356 = VISA Read(VISA resource name=w429, byte count=u32 6) -> (read buffer=w428:string)  [unwired: 1 in, 3 out]
                                n357 = local write "AutoStart ACK"(w428) -> ()
                              }
                            }
                          }
                          frame #4 {
                            n358 = while {
                              stop <- w431 stop-if-true
                              n359 = flat-sequence {
                                frame #0 {
                                w433 = "HM\u0015\u0000\u0000ª"  # AutoStart NACK
                                w434 = "HM211)"  # AutoStart
                                n360 = local read "AutoStart ACK"() -> (w432:string)
                                n361 = local read "COM Port"() -> (w435:refnum<visa-resource-name>)
                                n362 = Equal?(x=w432, y=w434) -> (x = y?=w437:bool)
                                n363 = Equal?(x=w432, y=w433) -> (x = y?=w436:bool)
                                n364 = case shown="True" w437 {
                                tunnel: w436 -> [w440 _]
                                tunnel: w435 -> [w439 _]
                                tunnel: w434 -> [w438 _]
                                frame False {
                                n365 = case shown="False" w440 {
                                tunnel: w439 -> [w442 w445]
                                tunnel: w438 -> [w441 w444]
                                frame False {
                                n366 = local write "WashACK"(FALSE ("WashACK")) -> ()
                                n367 = VISA Write(VISA resource name=w442, write buffer=w441) -> ()  [unwired: 1 in, 3 out]
                                }
                                frame True {
                                n368 = local write "WashACK"(FALSE ("WashACK")) -> ()
                                n369 = VISA Write(VISA resource name=w445, write buffer=w444) -> ()  [unwired: 1 in, 3 out]
                                }
                                }
                                }
                                frame True {
                                n370 = local write "WashACK"(TRUE ("WashACK")) -> ()
                                }
                                }
                                }
                                frame #1 {
                                n371 = local read "COM Port"() -> (w448:refnum<visa-resource-name>)
                                n372 = VISA Flush I/O Buffer(VISA resource name=w448) -> ()  [unwired: 1 in, 3 out]
                                }
                              }
                              n373 = local read "AUTO/STRT ACK"() -> (w431:bool)
                            }
                          }
                        }
                        "Autostart Ind" <- w405
                      }
                    }
                  }
                  frame Disabled {
                  }
                }
              }
              event "Wash": Value Change {
                w450 = i8 65 items=["Syringe"=83, "Temp"=84, "Pump"=80, "Walve "=86, "LED "=76, "JIG "=74, "Wash"=65, "Injection"=66, "Capture"=67, "Readout"=68]  # Commands
                n374 = event-data() -> ()  [unwired: 7 out]
                n375 = local write "WashACK"(FALSE ("WashACK")) -> ()
                n376 = local write "Commands"(w450) -> ()
                n377 = case shown="False" "Wash" {
                  selector: "Wash" -> [w452 w500]
                  frame False {
                    n378 = local write "Wash Ind"(w452) -> ()
                    n379 = stacked-sequence {
                      tunnel: [_ _ _ w462 _] -> _
                      frame #0 {
                        n380 = local read "COM Port"() -> (w453:refnum<visa-resource-name>)
                        n381 = VISA Flush I/O Buffer(VISA resource name=w453) -> ()  [unwired: 1 in, 3 out]
                      }
                      frame #1 {
                        w454 = i8 48 items=["STOP"=48, "Begin"=49]  # DATAs  Control
                        n382 = local write "DATAs\nControl"(w454) -> ()
                      }
                      frame #2 {
                        w457 = i8 49 items=["Write Command"=49]  # DATAs Command
                        w458 = i8 50  # Data Length
                        w460 = i8 72  # Header
                        n383 = local read "DATAs\nControl"() -> (w455:i8)
                        n384 = local read "Commands"() -> (w459:i8)
                        n385 = Compound Arithmetic op=ADD(w460, w459, w458, w457, w455) -> (w456:i8)
                        n386 = local write "Checksum"(w456) -> ()
                      }
                      frame #3 {
                        n387 = flat-sequence {
                          tunnel: [w463] -> w461
                          tunnel: [w480] -> w462
                          tunnel: w461 -> [w480]
                          frame #0 {
                            w475 = i8 50  # Data Length
                            w476 = i8 72  # Header
                            w474 = i8 49 items=["Write Command"=49]  # DATAs Command
                            n388 = local read "DATAs\nControl"() -> (w472:i8)
                            n389 = local read "Commands"() -> (w473:i8)
                            n390 = local read "Checksum"() -> (w471:i8)
                            n391 = Type Cast(x=w476) -> (*(type *) &x=w470:string)  [unwired: 1 out]
                            n392 = Type Cast(x=w471) -> (*(type *) &x=w465:string)  [unwired: 1 out]
                            n393 = Type Cast(x=w474) -> (*(type *) &x=w467:string)  [unwired: 1 out]
                            n394 = Type Cast(x=w472) -> (*(type *) &x=w466:string)  [unwired: 1 out]
                            n395 = Type Cast(x=w473) -> (*(type *) &x=w469:string)  [unwired: 1 out]
                            n396 = Type Cast(x=w475) -> (*(type *) &x=w468:string)  [unwired: 1 out]
                            n397 = Concatenate Strings(w470, w469, w468, w467, w466, w465) -> (w463:string)
                            n398 = local read "COM Port"() -> (w464:refnum<visa-resource-name>)
                            n399 = VISA Write(VISA resource name=w464, write buffer=w463) -> ()  [unwired: 1 in, 3 out]
                          }
                          frame #1 {
                            n400 = local read "COM Port"() -> (w478:refnum<visa-resource-name>)
                            n401 = VISA Read(VISA resource name=w478, byte count=u32 6) -> (read buffer=w477:string)  [unwired: 1 in, 3 out]
                            n402 = local write "Wash ACK"(w477) -> ()
                          }
                        }
                      }
                      frame #4 {
                        n403 = while {
                          stop <- w481 stop-if-true
                          n404 = flat-sequence {
                            frame #0 {
                              w486 = "HA\u0015\u0000\u0000ž"  # NACK
                              w484 = "HA210\u001c"  # Wash End
                              n405 = local read "Wash ACK"() -> (w483:string)
                              n406 = local read "COM Port"() -> (w482:refnum<visa-resource-name>)
                              n407 = Equal?(x=w483, y=w484) -> (x = y?=w487:bool)
                              n408 = Equal?(x=w483, y=w486) -> (x = y?=w485:bool)
                              n409 = case shown="True" w487 {
                                tunnel: w485 -> [w490 _]
                                tunnel: w482 -> [w489 _]
                                tunnel: w484 -> [w488 _]
                                frame False {
                                n410 = case shown="False" w490 {
                                tunnel: w489 -> [w492 w495]
                                tunnel: w488 -> [w491 w494]
                                frame False {
                                n411 = local write "WashACK"(FALSE ("WashACK")) -> ()
                                n412 = VISA Write(VISA resource name=w492, write buffer=w491) -> ()  [unwired: 1 in, 3 out]
                                }
                                frame True {
                                n413 = local write "WashACK"(FALSE ("WashACK")) -> ()
                                n414 = VISA Write(VISA resource name=w495, write buffer=w494) -> ()  [unwired: 1 in, 3 out]
                                }
                                }
                                }
                                frame True {
                                n415 = local write "WashACK"(TRUE ("WashACK")) -> ()
                                }
                              }
                            }
                            frame #1 {
                              n416 = local read "COM Port"() -> (w498:refnum<visa-resource-name>)
                              n417 = VISA Flush I/O Buffer(VISA resource name=w498) -> ()  [unwired: 1 in, 3 out]
                            }
                          }
                          n418 = local read "WashACK"() -> (w481:bool)
                        }
                      }
                    }
                  }
                  frame True {
                    w499 = FALSE ("Injection")
                    n419 = local write "Syringe Back"(w499) -> ()
                    n420 = local write "Syringe Ind"(w499) -> ()
                    n421 = local write "Injection"(w499) -> ()
                    n422 = local write "capture"(w499) -> ()
                    n423 = local write "Inj Ind"(w499) -> ()
                    n424 = local write "Cap Ind"(w499) -> ()
                    n425 = stacked-sequence {
                      frame #0 {
                        n426 = local read "COM Port"() -> (w501:refnum<visa-resource-name>)
                        n427 = VISA Flush I/O Buffer(VISA resource name=w501) -> ()  [unwired: 1 in, 3 out]
                      }
                      frame #1 {
                        w502 = i8 49 items=["STOP"=48, "Begin"=49]  # DATAs  Control
                        n428 = local write "DATAs\nControl"(w502) -> ()
                      }
                      frame #2 {
                        w506 = i8 49 items=["Write Command"=49]  # DATAs Command
                        w507 = i8 50  # Data Length
                        w508 = i8 72  # Header
                        n429 = local read "Commands"() -> (w505:i8)
                        n430 = local read "DATAs\nControl"() -> (w504:i8)
                        n431 = Compound Arithmetic op=ADD(w508, w505, w507, w506, w504) -> (w503:i8)
                        n432 = local write "Checksum"(w503) -> ()
                      }
                      frame #3 {
                        n433 = flat-sequence {
                          frame #0 {
                            w521 = i8 50  # Data Length
                            w522 = i8 72  # Header
                            w520 = i8 49 items=["Write Command"=49]  # DATAs Command
                            n434 = local read "DATAs\nControl"() -> (w512:i8)
                            n435 = local read "Commands"() -> (w511:i8)
                            n436 = local read "Checksum"() -> (w513:i8)
                            n437 = Type Cast(x=w522) -> (*(type *) &x=w519:string)  [unwired: 1 out]
                            n438 = Type Cast(x=w511) -> (*(type *) &x=w518:string)  [unwired: 1 out]
                            n439 = Type Cast(x=w513) -> (*(type *) &x=w514:string)  [unwired: 1 out]
                            n440 = Type Cast(x=w520) -> (*(type *) &x=w516:string)  [unwired: 1 out]
                            n441 = Type Cast(x=w512) -> (*(type *) &x=w515:string)  [unwired: 1 out]
                            n442 = Type Cast(x=w521) -> (*(type *) &x=w517:string)  [unwired: 1 out]
                            n443 = Concatenate Strings(w519, w518, w517, w516, w515, w514) -> (w509:string)
                            n444 = local read "COM Port"() -> (w510:refnum<visa-resource-name>)
                            n445 = VISA Write(VISA resource name=w510, write buffer=w509) -> ()  [unwired: 1 in, 3 out]
                          }
                          frame #1 {
                            n446 = local read "COM Port"() -> (w524:refnum<visa-resource-name>)
                            n447 = VISA Read(VISA resource name=w524, byte count=u32 6) -> (read buffer=w523:string)  [unwired: 1 in, 3 out]
                            n448 = local write "Wash ACK"(w523) -> ()
                          }
                        }
                      }
                      frame #4 {
                        n449 = while {
                          stop <- w526 stop-if-true
                          n450 = flat-sequence {
                            frame #0 {
                              w531 = "HA\u0015\u0000\u0000ž"  # NACK
                              w529 = "HA211\u001d"  # Wash Begin
                              n451 = local read "Wash ACK"() -> (w528:string)
                              n452 = local read "COM Port"() -> (w527:refnum<visa-resource-name>)
                              n453 = Equal?(x=w528, y=w529) -> (x = y?=w532:bool)
                              n454 = Equal?(x=w528, y=w531) -> (x = y?=w530:bool)
                              n455 = case shown="True" w532 {
                                tunnel: w530 -> [w535 _]
                                tunnel: w527 -> [w534 _]
                                tunnel: w529 -> [w533 _]
                                frame False {
                                n456 = case shown="False" w535 {
                                tunnel: w534 -> [w537 w540]
                                tunnel: w533 -> [w536 w539]
                                frame False {
                                n457 = local write "WashACK"(FALSE ("WashACK")) -> ()
                                n458 = VISA Write(VISA resource name=w537, write buffer=w536) -> ()  [unwired: 1 in, 3 out]
                                }
                                frame True {
                                n459 = local write "WashACK"(FALSE ("WashACK")) -> ()
                                n460 = VISA Write(VISA resource name=w540, write buffer=w539) -> ()  [unwired: 1 in, 3 out]
                                }
                                }
                                }
                                frame True {
                                n461 = local write "WashACK"(TRUE ("WashACK")) -> ()
                                }
                              }
                            }
                            frame #1 {
                              n462 = local read "COM Port"() -> (w543:refnum<visa-resource-name>)
                              n463 = VISA Flush I/O Buffer(VISA resource name=w543) -> ()  [unwired: 1 in, 3 out]
                            }
                          }
                          n464 = local read "WashACK"() -> (w526:bool)
                        }
                      }
                    }
                    "Wash Ind" <- w500
                  }
                }
              }
              event "Injection": Value Change {
                w545 = i8 66 items=["Syringe"=83, "Temp"=84, "Pump"=80, "Walve "=86, "LED "=76, "JIG "=74, "Wash"=65, "Injection"=66, "Capture"=67, "Readout"=68]  # Commands
                n465 = event-data() -> ()  [unwired: 7 out]
                n466 = local write "Inj ACK"(FALSE ("Inj ACK")) -> ()
                n467 = local write "Commands"(w545) -> ()
                n468 = case shown="True" "Injection" {
                  selector: "Injection" -> [w547 w592]
                  frame False {
                    n469 = local write "Inj Ind"(w547) -> ()
                    n470 = stacked-sequence {
                      frame #0 {
                        n471 = local read "COM Port"() -> (w548:refnum<visa-resource-name>)
                        n472 = VISA Flush I/O Buffer(VISA resource name=w548) -> ()  [unwired: 1 in, 3 out]
                      }
                      frame #1 {
                        w549 = i8 48 items=["STOP"=48, "Begin"=49]  # DATAs  Control
                        n473 = local write "DATAs\nControl"(w549) -> ()
                      }
                      frame #2 {
                        w553 = i8 49 items=["Write Command"=49]  # DATAs Command
                        w554 = i8 50  # Data Length
                        w555 = i8 72  # Header
                        n474 = local read "Commands"() -> (w552:i8)
                        n475 = local read "DATAs\nControl"() -> (w551:i8)
                        n476 = Compound Arithmetic op=ADD(w555, w552, w554, w553, w551) -> (w550:i8)
                        n477 = local write "Checksum"(w550) -> ()
                      }
                      frame #3 {
                        n478 = flat-sequence {
                          frame #0 {
                            w561 = i8 50  # Data Length
                            w569 = i8 72  # Header
                            w568 = i8 49 items=["Write Command"=49]  # DATAs Command
                            n479 = local read "DATAs\nControl"() -> (w559:i8)
                            n480 = local read "Commands"() -> (w560:i8)
                            n481 = local read "Checksum"() -> (w558:i8)
                            n482 = Type Cast(x=w569) -> (*(type *) &x=w567:string)  [unwired: 1 out]
                            n483 = Type Cast(x=w558) -> (*(type *) &x=w562:string)  [unwired: 1 out]
                            n484 = Type Cast(x=w568) -> (*(type *) &x=w564:string)  [unwired: 1 out]
                            n485 = Type Cast(x=w559) -> (*(type *) &x=w563:string)  [unwired: 1 out]
                            n486 = Type Cast(x=w560) -> (*(type *) &x=w566:string)  [unwired: 1 out]
                            n487 = Type Cast(x=w561) -> (*(type *) &x=w565:string)  [unwired: 1 out]
                            n488 = Concatenate Strings(w567, w566, w565, w564, w563, w562) -> (w556:string)
                            n489 = local read "COM Port"() -> (w557:refnum<visa-resource-name>)
                            n490 = VISA Write(VISA resource name=w557, write buffer=w556) -> ()  [unwired: 1 in, 3 out]
                          }
                          frame #1 {
                            n491 = local read "COM Port"() -> (w572:refnum<visa-resource-name>)
                            n492 = VISA Read(VISA resource name=w572, byte count=u32 6) -> (read buffer=w570:string)  [unwired: 1 in, 3 out]
                            n493 = local write "Injection ACK"(w570) -> ()
                          }
                        }
                      }
                      frame #4 {
                        n494 = while {
                          stop <- w573 stop-if-true
                          n495 = flat-sequence {
                            frame #0 {
                              w576 = "HB210\u001d"  # Injection End
                              w578 = "HB\u0015\u0000\u0000Ÿ"  # Injection NACK
                              n496 = local read "Injection ACK"() -> (w574:string)
                              n497 = local read "COM Port"() -> (w575:refnum<visa-resource-name>)
                              n498 = Equal?(x=w574, y=w576) -> (x = y?=w579:bool)
                              n499 = Equal?(x=w574, y=w578) -> (x = y?=w577:bool)
                              n500 = case shown="False" w579 {
                                tunnel: w577 -> [w582 _]
                                tunnel: w575 -> [w581 _]
                                tunnel: w576 -> [w580 _]
                                frame False {
                                n501 = case shown="False" w582 {
                                tunnel: w581 -> [w584 w587]
                                tunnel: w580 -> [w583 w586]
                                frame False {
                                n502 = local write "Inj ACK"(FALSE ("Inj ACK")) -> ()
                                n503 = VISA Write(VISA resource name=w584, write buffer=w583) -> ()  [unwired: 1 in, 3 out]
                                }
                                frame True {
                                n504 = local write "Inj ACK"(FALSE ("Inj ACK")) -> ()
                                n505 = VISA Write(VISA resource name=w587, write buffer=w586) -> ()  [unwired: 1 in, 3 out]
                                }
                                }
                                }
                                frame True {
                                n506 = local write "Inj ACK"(TRUE ("Inj ACK")) -> ()
                                }
                              }
                            }
                            frame #1 {
                              n507 = local read "COM Port"() -> (w590:refnum<visa-resource-name>)
                              n508 = VISA Flush I/O Buffer(VISA resource name=w590) -> ()  [unwired: 1 in, 3 out]
                            }
                          }
                          n509 = local read "Inj ACK"() -> (w573:bool)
                        }
                      }
                    }
                  }
                  frame True {
                    w591 = FALSE ("capture")
                    n510 = local write "Syringe Ind"(w591) -> ()
                    n511 = local write "Wash"(w591) -> ()
                    n512 = local write "Syringe Back"(w591) -> ()
                    n513 = local write "capture"(w591) -> ()
                    n514 = local write "Cap Ind"(w591) -> ()
                    n515 = local write "Wash Ind"(w591) -> ()
                    n516 = stacked-sequence {
                      frame #0 {
                        n517 = local read "COM Port"() -> (w593:refnum<visa-resource-name>)
                        n518 = VISA Flush I/O Buffer(VISA resource name=w593) -> ()  [unwired: 1 in, 3 out]
                      }
                      frame #1 {
                        w594 = i8 49 items=["STOP"=48, "Begin"=49]  # DATAs  Control
                        n519 = local write "DATAs\nControl"(w594) -> ()
                      }
                      frame #2 {
                        w598 = i8 49 items=["Write Command"=49]  # DATAs Command
                        w599 = i8 50  # Data Length
                        w600 = i8 72  # Header
                        n520 = local read "Commands"() -> (w597:i8)
                        n521 = local read "DATAs\nControl"() -> (w596:i8)
                        n522 = Compound Arithmetic op=ADD(w600, w597, w599, w598, w596) -> (w595:i8)
                        n523 = local write "Checksum"(w595) -> ()
                      }
                      frame #3 {
                        n524 = flat-sequence {
                          frame #0 {
                            w606 = i8 50  # Data Length
                            w614 = i8 72  # Header
                            w613 = i8 49 items=["Write Command"=49]  # DATAs Command
                            n525 = local read "Commands"() -> (w605:i8)
                            n526 = local read "DATAs\nControl"() -> (w604:i8)
                            n527 = local read "Checksum"() -> (w603:i8)
                            n528 = Type Cast(x=w614) -> (*(type *) &x=w612:string)  [unwired: 1 out]
                            n529 = Type Cast(x=w603) -> (*(type *) &x=w607:string)  [unwired: 1 out]
                            n530 = Type Cast(x=w613) -> (*(type *) &x=w609:string)  [unwired: 1 out]
                            n531 = Type Cast(x=w604) -> (*(type *) &x=w608:string)  [unwired: 1 out]
                            n532 = Type Cast(x=w605) -> (*(type *) &x=w611:string)  [unwired: 1 out]
                            n533 = Type Cast(x=w606) -> (*(type *) &x=w610:string)  [unwired: 1 out]
                            n534 = Concatenate Strings(w612, w611, w610, w609, w608, w607) -> (w601:string)
                            n535 = local read "COM Port"() -> (w602:refnum<visa-resource-name>)
                            n536 = VISA Write(VISA resource name=w602, write buffer=w601) -> ()  [unwired: 1 in, 3 out]
                          }
                          frame #1 {
                            n537 = local read "COM Port"() -> (w617:refnum<visa-resource-name>)
                            n538 = VISA Read(VISA resource name=w617, byte count=u32 6) -> (read buffer=w615:string)  [unwired: 1 in, 3 out]
                            n539 = local write "Injection ACK"(w615) -> ()
                          }
                        }
                      }
                      frame #4 {
                        n540 = while {
                          stop <- w618 stop-if-true
                          n541 = flat-sequence {
                            frame #0 {
                              w619 = "HB211\u001e"  # Injection Begin
                              w623 = "HB\u0015\u0000\u0000Ÿ"  # Injection NACK
                              n542 = local read "Injection ACK"() -> (w620:string)
                              n543 = local read "COM Port"() -> (w621:refnum<visa-resource-name>)
                              n544 = Equal?(x=w620, y=w619) -> (x = y?=w624:bool)
                              n545 = Equal?(x=w620, y=w623) -> (x = y?=w622:bool)
                              n546 = case shown="False" w624 {
                                tunnel: w622 -> [w627 _]
                                tunnel: w621 -> [w626 _]
                                tunnel: w619 -> [w625 _]
                                frame False {
                                n547 = case shown="False" w627 {
                                tunnel: w626 -> [w629 w632]
                                tunnel: w625 -> [w628 w631]
                                frame False {
                                n548 = local write "Inj ACK"(FALSE ("Inj ACK")) -> ()
                                n549 = VISA Write(VISA resource name=w629, write buffer=w628) -> ()  [unwired: 1 in, 3 out]
                                }
                                frame True {
                                n550 = local write "Inj ACK"(FALSE ("Inj ACK")) -> ()
                                n551 = VISA Write(VISA resource name=w632, write buffer=w631) -> ()  [unwired: 1 in, 3 out]
                                }
                                }
                                }
                                frame True {
                                n552 = local write "Inj ACK"(TRUE ("Inj ACK")) -> ()
                                }
                              }
                            }
                            frame #1 {
                              n553 = local read "COM Port"() -> (w635:refnum<visa-resource-name>)
                              n554 = VISA Flush I/O Buffer(VISA resource name=w635) -> ()  [unwired: 1 in, 3 out]
                            }
                          }
                          n555 = local read "Inj ACK"() -> (w618:bool)
                        }
                      }
                    }
                    "Inj Ind" <- w592
                  }
                }
              }
              event "capture": Value Change {
                w638 = i8 67 items=["Syringe"=83, "Temp"=84, "Pump"=80, "Walve "=86, "LED "=76, "JIG "=74, "Wash"=65, "Injection"=66, "Capture"=67, "Readout"=68]  # Commands
                n556 = event-data() -> ()  [unwired: 7 out]
                n557 = global write "Image Acq..vi" "Image Acq."("capture") -> ()
                n558 = local write "Commands"(w638) -> ()
                n559 = local write "CAP ACK"(FALSE ("CAP ACK")) -> ()
                n560 = case shown="True" "capture" {
                  selector: "capture" -> [w639 w684]
                  frame False {
                    n561 = local write "Cap Ind"(w639) -> ()
                    n562 = stacked-sequence {
                      frame #0 {
                        n563 = local read "COM Port"() -> (w640:refnum<visa-resource-name>)
                        n564 = VISA Flush I/O Buffer(VISA resource name=w640) -> ()  [unwired: 1 in, 3 out]
                      }
                      frame #1 {
                        w641 = i8 48 items=["STOP"=48, "Begin"=49]  # DATAs  Control
                        n565 = local write "DATAs\nControl"(w641) -> ()
                      }
                      frame #2 {
                        w644 = i8 49 items=["Write Command"=49]  # DATAs Command
                        w643 = i8 50  # Data Length
                        w642 = i8 72  # Header
                        n566 = local read "Commands"() -> (w645:i8)
                        n567 = local read "DATAs\nControl"() -> (w646:i8)
                        n568 = Compound Arithmetic op=ADD(w642, w645, w643, w644, w646) -> (w647:i8)
                        n569 = local write "Checksum"(w647) -> ()
                      }
                      frame #3 {
                        n570 = flat-sequence {
                          frame #0 {
                            w657 = i8 50  # Data Length
                            w648 = i8 72  # Header
                            w649 = i8 49 items=["Write Command"=49]  # DATAs Command
                            n571 = local read "DATAs\nControl"() -> (w659:i8)
                            n572 = local read "Commands"() -> (w658:i8)
                            n573 = local read "Checksum"() -> (w656:i8)
                            n574 = Type Cast(x=w648) -> (*(type *) &x=w650:string)  [unwired: 1 out]
                            n575 = Type Cast(x=w656) -> (*(type *) &x=w655:string)  [unwired: 1 out]
                            n576 = Type Cast(x=w649) -> (*(type *) &x=w653:string)  [unwired: 1 out]
                            n577 = Type Cast(x=w659) -> (*(type *) &x=w654:string)  [unwired: 1 out]
                            n578 = Type Cast(x=w658) -> (*(type *) &x=w651:string)  [unwired: 1 out]
                            n579 = Type Cast(x=w657) -> (*(type *) &x=w652:string)  [unwired: 1 out]
                            n580 = Concatenate Strings(w650, w651, w652, w653, w654, w655) -> (w661:string)
                            n581 = local read "COM Port"() -> (w660:refnum<visa-resource-name>)
                            n582 = VISA Write(VISA resource name=w660, write buffer=w661) -> ()  [unwired: 1 in, 3 out]
                          }
                          frame #1 {
                            n583 = local read "COM Port"() -> (w664:refnum<visa-resource-name>)
                            n584 = VISA Read(VISA resource name=w664, byte count=u32 6) -> (read buffer=w662:string)  [unwired: 1 in, 3 out]
                            n585 = local write "Capture ACK"(w662) -> ()
                          }
                        }
                      }
                      frame #4 {
                        n586 = while {
                          stop <- w665 stop-if-true
                          n587 = flat-sequence {
                            frame #0 {
                              w666 = "HC210\u001e"  # Capture End
                              w670 = "HC\u0015\u0000\u0000 "  # Capture NACK
                              n588 = local read "Capture ACK"() -> (w667:string)
                              n589 = local read "COM Port"() -> (w668:refnum<visa-resource-name>)
                              n590 = Equal?(x=w667, y=w666) -> (x = y?=w671:bool)
                              n591 = Equal?(x=w667, y=w670) -> (x = y?=w669:bool)
                              n592 = case shown="False" w671 {
                                tunnel: w669 -> [w674 _]
                                tunnel: w668 -> [w673 _]
                                tunnel: w666 -> [w672 _]
                                frame False {
                                n593 = case shown="False" w674 {
                                tunnel: w673 -> [w676 w679]
                                tunnel: w672 -> [w675 w678]
                                frame False {
                                n594 = local write "CAP ACK"(FALSE ("CAP ACK")) -> ()
                                n595 = VISA Write(VISA resource name=w676, write buffer=w675) -> ()  [unwired: 1 in, 3 out]
                                }
                                frame True {
                                n596 = local write "CAP ACK"(FALSE ("CAP ACK")) -> ()
                                n597 = VISA Write(VISA resource name=w679, write buffer=w678) -> ()  [unwired: 1 in, 3 out]
                                }
                                }
                                }
                                frame True {
                                n598 = local write "CAP ACK"(TRUE ("CAP ACK")) -> ()
                                }
                              }
                            }
                            frame #1 {
                              n599 = local read "COM Port"() -> (w682:refnum<visa-resource-name>)
                              n600 = VISA Flush I/O Buffer(VISA resource name=w682) -> ()  [unwired: 1 in, 3 out]
                            }
                          }
                          n601 = local read "CAP ACK"() -> (w665:bool)
                        }
                      }
                      frame #5 {
                        n602 = local read "IMAQ USB Session Out 2"() -> (w683:T2)
                        n603 = call <vilib>:"IMAQ USB Grab Setup.vi"("IMAQ USB Session In"=w683) -> ()  [unwired: 1 in, 10 out]
                      }
                    }
                  }
                  frame True {
                    w685 = FALSE ("Read Ind")
                    n604 = local write "Wash"(w685) -> ()
                    n605 = local write "Syringe Ind"(w685) -> ()
                    n606 = local write "Syringe Back"(w685) -> ()
                    n607 = local write "Wash Ind"(w685) -> ()
                    n608 = local write "Injection"(w685) -> ()
                    n609 = local write "Inj Ind"(w685) -> ()
                    n610 = stacked-sequence {
                      frame #0 {
                        n611 = local read "COM Port"() -> (w686:refnum<visa-resource-name>)
                        n612 = VISA Flush I/O Buffer(VISA resource name=w686) -> ()  [unwired: 1 in, 3 out]
                      }
                      frame #1 {
                        w687 = i8 49 items=["STOP"=48, "Begin"=49]  # DATAs  Control
                        n613 = local write "DATAs\nControl"(w687) -> ()
                      }
                      frame #2 {
                        w690 = i8 49 items=["Write Command"=49]  # DATAs Command
                        w692 = i8 50  # Data Length
                        w693 = i8 72  # Header
                        n614 = local read "Commands"() -> (w691:i8)
                        n615 = local read "DATAs\nControl"() -> (w689:i8)
                        n616 = Compound Arithmetic op=ADD(w693, w691, w692, w690, w689) -> (w688:i8)
                        n617 = local write "Checksum"(w688) -> ()
                      }
                      frame #3 {
                        n618 = flat-sequence {
                          frame #0 {
                            w706 = i8 50  # Data Length
                            w707 = i8 72  # Header
                            w705 = i8 49 items=["Write Command"=49]  # DATAs Command
                            n619 = local read "Commands"() -> (w698:i8)
                            n620 = local read "DATAs\nControl"() -> (w696:i8)
                            n621 = local read "Checksum"() -> (w697:i8)
                            n622 = Type Cast(x=w707) -> (*(type *) &x=w704:string)  [unwired: 1 out]
                            n623 = Type Cast(x=w697) -> (*(type *) &x=w699:string)  [unwired: 1 out]
                            n624 = Type Cast(x=w705) -> (*(type *) &x=w701:string)  [unwired: 1 out]
                            n625 = Type Cast(x=w696) -> (*(type *) &x=w700:string)  [unwired: 1 out]
                            n626 = Type Cast(x=w698) -> (*(type *) &x=w703:string)  [unwired: 1 out]
                            n627 = Type Cast(x=w706) -> (*(type *) &x=w702:string)  [unwired: 1 out]
                            n628 = Concatenate Strings(w704, w703, w702, w701, w700, w699) -> (w694:string)
                            n629 = local read "COM Port"() -> (w695:refnum<visa-resource-name>)
                            n630 = VISA Write(VISA resource name=w695, write buffer=w694) -> ()  [unwired: 1 in, 3 out]
                          }
                          frame #1 {
                            n631 = local read "COM Port"() -> (w710:refnum<visa-resource-name>)
                            n632 = VISA Read(VISA resource name=w710, byte count=u32 6) -> (read buffer=w708:string)  [unwired: 1 in, 3 out]
                            n633 = local write "Capture ACK"(w708) -> ()
                          }
                        }
                      }
                      frame #4 {
                        n634 = while {
                          stop <- w711 stop-if-true
                          n635 = flat-sequence {
                            frame #0 {
                              w716 = "HC\u0015\u0000\u0000 "  # Capture NACK
                              w714 = "HC211\u001f"  # Capture Begin
                              n636 = local read "Capture ACK"() -> (w712:string)
                              n637 = local read "COM Port"() -> (w713:refnum<visa-resource-name>)
                              n638 = Equal?(x=w712, y=w714) -> (x = y?=w717:bool)
                              n639 = Equal?(x=w712, y=w716) -> (x = y?=w715:bool)
                              n640 = case shown="False" w717 {
                                tunnel: w715 -> [w720 _]
                                tunnel: w713 -> [w719 _]
                                tunnel: w714 -> [w718 _]
                                frame False {
                                n641 = case shown="False" w720 {
                                tunnel: w719 -> [w722 w725]
                                tunnel: w718 -> [w721 w724]
                                frame False {
                                n642 = local write "CAP ACK"(FALSE ("CAP ACK")) -> ()
                                n643 = VISA Write(VISA resource name=w722, write buffer=w721) -> ()  [unwired: 1 in, 3 out]
                                }
                                frame True {
                                n644 = local write "CAP ACK"(FALSE ("CAP ACK")) -> ()
                                n645 = VISA Write(VISA resource name=w725, write buffer=w724) -> ()  [unwired: 1 in, 3 out]
                                }
                                }
                                }
                                frame True {
                                n646 = local write "CAP ACK"(TRUE ("CAP ACK")) -> ()
                                }
                              }
                            }
                            frame #1 {
                              n647 = local read "COM Port"() -> (w728:refnum<visa-resource-name>)
                              n648 = VISA Flush I/O Buffer(VISA resource name=w728) -> ()  [unwired: 1 in, 3 out]
                            }
                          }
                          n649 = local read "CAP ACK"() -> (w711:bool)
                        }
                      }
                      frame #5 {
                        n650 = local read "IMAQ USB Session Out 2"() -> (w730:T2)
                        n651 = local read "Image"() -> (w732:T1)
                        n652 = call <vilib>:"IMAQ USB Snap.vi"("Image in"=w732, "IMAQ USB Session In"=w730) -> ("Image out"=w733:T1)  [unwired: 1 in, 8 out]
                        n653 = call-poly "IMAQ Write File 2"("File Path"="Image File Path (jpg)", "Image"=w733) -> ("Image Out (duplicate)"=→"Image Out (duplicate)":T1)  [unwired: 3 in, 6 out]
                      }
                    }
                    "Cap Ind" <- w684
                  }
                }
              }
              event "Syringe Back": Value Change {
                w735 = i8 68 items=["Syringe"=83, "Temp"=84, "Pump"=80, "Walve "=86, "LED "=76, "JIG "=74, "Wash"=65, "Injection"=66, "Capture"=67, "Readout"=68]  # Commands
                n654 = event-data() -> ()  [unwired: 7 out]
                n655 = local write "SYRINGE ACK"(FALSE ("SYRINGE ACK")) -> ()
                n656 = local write "Commands"(w735) -> ()
                n657 = case shown="False" "Syringe Back" {
                  selector: "Syringe Back" -> [w737 w782]
                  frame False {
                    n658 = local write "Syringe Ind"(w737) -> ()
                    n659 = stacked-sequence {
                      frame #0 {
                        n660 = local read "COM Port"() -> (w738:refnum<visa-resource-name>)
                        n661 = VISA Flush I/O Buffer(VISA resource name=w738) -> ()  [unwired: 1 in, 3 out]
                      }
                      frame #1 {
                        w739 = i8 48 items=["STOP"=48, "Begin"=49]  # DATAs  Control
                        n662 = local write "DATAs\nControl"(w739) -> ()
                      }
                      frame #2 {
                        w743 = i8 49 items=["Write Command"=49]  # DATAs Command
                        w744 = i8 50  # Data Length
                        w745 = i8 72  # Header
                        n663 = local read "DATAs\nControl"() -> (w741:i8)
                        n664 = local read "Commands"() -> (w742:i8)
                        n665 = Compound Arithmetic op=ADD(w745, w742, w744, w743, w741) -> (w740:i8)
                        n666 = local write "Checksum"(w740) -> ()
                      }
                      frame #3 {
                        n667 = flat-sequence {
                          frame #0 {
                            w758 = i8 50  # Data Length
                            w759 = i8 72  # Header
                            w757 = i8 49 items=["Write Command"=49]  # DATAs Command
                            n668 = local read "DATAs\nControl"() -> (w749:i8)
                            n669 = local read "Checksum"() -> (w748:i8)
                            n670 = local read "Commands"() -> (w750:i8)
                            n671 = Type Cast(x=w759) -> (*(type *) &x=w756:string)  [unwired: 1 out]
                            n672 = Type Cast(x=w748) -> (*(type *) &x=w751:string)  [unwired: 1 out]
                            n673 = Type Cast(x=w757) -> (*(type *) &x=w753:string)  [unwired: 1 out]
                            n674 = Type Cast(x=w749) -> (*(type *) &x=w752:string)  [unwired: 1 out]
                            n675 = Type Cast(x=w750) -> (*(type *) &x=w755:string)  [unwired: 1 out]
                            n676 = Type Cast(x=w758) -> (*(type *) &x=w754:string)  [unwired: 1 out]
                            n677 = Concatenate Strings(w756, w755, w754, w753, w752, w751) -> (w746:string)
                            n678 = local read "COM Port"() -> (w747:refnum<visa-resource-name>)
                            n679 = VISA Write(VISA resource name=w747, write buffer=w746) -> ()  [unwired: 1 in, 3 out]
                          }
                          frame #1 {
                            n680 = local read "COM Port"() -> (w762:refnum<visa-resource-name>)
                            n681 = VISA Read(VISA resource name=w762, byte count=u32 6) -> (read buffer=w760:string)  [unwired: 1 in, 3 out]
                            n682 = local write "Syringe ACK"(w760) -> ()
                          }
                        }
                      }
                      frame #4 {
                        n683 = while {
                          stop <- w763 stop-if-true
                          n684 = flat-sequence {
                            frame #0 {
                              w764 = "HD210\u001f"  # Syringe Rel. End
                              w768 = "HD\u0015\u0000\u0000¡"  # Syringe Rel. NACK
                              n685 = local read "Syringe ACK"() -> (w765:string)
                              n686 = local read "COM Port"() -> (w766:refnum<visa-resource-name>)
                              n687 = Equal?(x=w765, y=w764) -> (x = y?=w769:bool)
                              n688 = Equal?(x=w765, y=w768) -> (x = y?=w767:bool)
                              n689 = case shown="False" w769 {
                                tunnel: w767 -> [w772 _]
                                tunnel: w766 -> [w771 _]
                                tunnel: w764 -> [w770 _]
                                frame False {
                                n690 = case shown="True" w772 {
                                tunnel: w771 -> [w775 w777]
                                tunnel: w770 -> [w774 w776]
                                frame False {
                                n691 = local write "SYRINGE ACK"(FALSE ("SYRINGE ACK")) -> ()
                                n692 = VISA Write(VISA resource name=w775, write buffer=w774) -> ()  [unwired: 1 in, 3 out]
                                }
                                frame True {
                                n693 = local write "SYRINGE ACK"(FALSE ("SYRINGE ACK")) -> ()
                                n694 = VISA Write(VISA resource name=w777, write buffer=w776) -> ()  [unwired: 1 in, 3 out]
                                }
                                }
                                }
                                frame True {
                                n695 = local write "SYRINGE ACK"(TRUE ("SYRINGE ACK")) -> ()
                                }
                              }
                            }
                            frame #1 {
                              n696 = local read "COM Port"() -> (w780:refnum<visa-resource-name>)
                              n697 = VISA Flush I/O Buffer(VISA resource name=w780) -> ()  [unwired: 1 in, 3 out]
                            }
                          }
                          n698 = local read "SYRINGE ACK"() -> (w763:bool)
                        }
                      }
                    }
                  }
                  frame True {
                    w781 = FALSE ("Wash Ind")
                    n699 = local write "Inj Ind"(w781) -> ()
                    n700 = local write "Injection"(w781) -> ()
                    n701 = local write "Wash"(w781) -> ()
                    n702 = local write "capture"(w781) -> ()
                    n703 = local write "Wash Ind"(w781) -> ()
                    n704 = local write "Cap Ind"(w781) -> ()
                    n705 = stacked-sequence {
                      frame #0 {
                        n706 = local read "COM Port"() -> (w783:refnum<visa-resource-name>)
                        n707 = VISA Flush I/O Buffer(VISA resource name=w783) -> ()  [unwired: 1 in, 3 out]
                      }
                      frame #1 {
                        w784 = i8 49 items=["STOP"=48, "Begin"=49]  # DATAs  Control
                        n708 = local write "DATAs\nControl"(w784) -> ()
                      }
                      frame #2 {
                        w788 = i8 49 items=["Write Command"=49]  # DATAs Command
                        w789 = i8 50  # Data Length
                        w790 = i8 72  # Header
                        n709 = local read "Commands"() -> (w787:i8)
                        n710 = local read "DATAs\nControl"() -> (w785:i8)
                        n711 = Compound Arithmetic op=ADD(w790, w787, w789, w788, w785) -> (w786:i8)
                        n712 = local write "Checksum"(w786) -> ()
                      }
                      frame #3 {
                        n713 = flat-sequence {
                          frame #0 {
                            w803 = i8 50  # Data Length
                            w804 = i8 72  # Header
                            w802 = i8 49 items=["Write Command"=49]  # DATAs Command
                            n714 = local read "DATAs\nControl"() -> (w794:i8)
                            n715 = local read "Commands"() -> (w795:i8)
                            n716 = local read "Checksum"() -> (w793:i8)
                            n717 = Type Cast(x=w804) -> (*(type *) &x=w801:string)  [unwired: 1 out]
                            n718 = Type Cast(x=w793) -> (*(type *) &x=w796:string)  [unwired: 1 out]
                            n719 = Type Cast(x=w802) -> (*(type *) &x=w798:string)  [unwired: 1 out]
                            n720 = Type Cast(x=w794) -> (*(type *) &x=w797:string)  [unwired: 1 out]
                            n721 = Type Cast(x=w795) -> (*(type *) &x=w800:string)  [unwired: 1 out]
                            n722 = Type Cast(x=w803) -> (*(type *) &x=w799:string)  [unwired: 1 out]
                            n723 = Concatenate Strings(w801, w800, w799, w798, w797, w796) -> (w791:string)
                            n724 = local read "COM Port"() -> (w792:refnum<visa-resource-name>)
                            n725 = VISA Write(VISA resource name=w792, write buffer=w791) -> ()  [unwired: 1 in, 3 out]
                          }
                          frame #1 {
                            n726 = local read "COM Port"() -> (w807:refnum<visa-resource-name>)
                            n727 = VISA Read(VISA resource name=w807, byte count=u32 6) -> (read buffer=w805:string)  [unwired: 1 in, 3 out]
                            n728 = local write "Syringe ACK"(w805) -> ()
                          }
                        }
                      }
                      frame #4 {
                        n729 = while {
                          stop <- w808 stop-if-true
                          n730 = flat-sequence {
                            frame #0 {
                              w813 = "HD\u0015\u0000\u0000¡"  # Syringe Rel. NACK
                              w811 = "HD211 "  # Syringe Rel. Begin
                              n731 = local read "Syringe ACK"() -> (w809:string)
                              n732 = local read "COM Port"() -> (w810:refnum<visa-resource-name>)
                              n733 = Equal?(x=w809, y=w811) -> (x = y?=w814:bool)
                              n734 = Equal?(x=w809, y=w813) -> (x = y?=w812:bool)
                              n735 = case shown="False" w814 {
                                tunnel: w812 -> [w817 _]
                                tunnel: w810 -> [w816 _]
                                tunnel: w811 -> [w815 _]
                                frame False {
                                n736 = case shown="True" w817 {
                                tunnel: w816 -> [w820 w822]
                                tunnel: w815 -> [w819 w821]
                                frame False {
                                n737 = local write "SYRINGE ACK"(FALSE ("SYRINGE ACK")) -> ()
                                n738 = VISA Write(VISA resource name=w820, write buffer=w819) -> ()  [unwired: 1 in, 3 out]
                                }
                                frame True {
                                n739 = local write "SYRINGE ACK"(FALSE ("SYRINGE ACK")) -> ()
                                n740 = VISA Write(VISA resource name=w822, write buffer=w821) -> ()  [unwired: 1 in, 3 out]
                                }
                                }
                                }
                                frame True {
                                n741 = local write "SYRINGE ACK"(TRUE ("SYRINGE ACK")) -> ()
                                }
                              }
                            }
                            frame #1 {
                              n742 = local read "COM Port"() -> (w825:refnum<visa-resource-name>)
                              n743 = VISA Flush I/O Buffer(VISA resource name=w825) -> ()  [unwired: 1 in, 3 out]
                            }
                          }
                          n744 = local read "SYRINGE ACK"() -> (w808:bool)
                        }
                      }
                    }
                    "Syringe Ind" <- w782
                  }
                }
              }
              event "Emergency\nStop": Value Change {
                n745 = event-data() -> ()  [unwired: 7 out]
                n746 = local write "EMER STOP ACK"(FALSE ("EMER STOP ACK")) -> ()
                n747 = case shown="True" "Emergency\nStop" {
                  frame False {
                  }
                  frame True {
                    n748 = stacked-sequence {
                      frame #0 {
                        n749 = local read "COM Port"() -> (w828:refnum<visa-resource-name>)
                        n750 = VISA Flush I/O Buffer(VISA resource name=w828) -> ()  [unwired: 1 in, 3 out]
                      }
                      frame #1 {
                        n751 = flat-sequence {
                          frame #0 {
                            n752 = local read "COM Port"() -> (w830:refnum<visa-resource-name>)
                            n753 = VISA Write(VISA resource name=w830, write buffer="HE11ï") -> ()  [unwired: 1 in, 3 out]
                          }
                          frame #1 {
                            n754 = local read "COM Port"() -> (w831:refnum<visa-resource-name>)
                            n755 = VISA Read(VISA resource name=w831, byte count=u32 5) -> (read buffer=w833:string)  [unwired: 1 in, 3 out]
                            n756 = local write "Emer Stop ACK"(w833) -> ()
                          }
                        }
                      }
                      frame #2 {
                        n757 = while {
                          stop <- w834 stop-if-true
                          n758 = flat-sequence {
                            frame #0 {
                              w839 = "HE\u0015\u0000\u0000¢"  # Emer Stop NACK
                              w838 = "HE11ï"  # Emergency Stop
                              n759 = local read "Emer Stop ACK"() -> (w835:string)
                              "Stop read buffer" <- w835
                              n760 = local read "COM Port"() -> (w836:refnum<visa-resource-name>)
                              n761 = Equal?(x=w835, y=w838) -> (x = y?=w840:bool)
                              n762 = Equal?(x=w835, y=w839) -> (x = y?=w837:bool)
                              n763 = case shown="False" w840 {
                                tunnel: w838 -> [w842 _]
                                tunnel: w836 -> [w843 _]
                                tunnel: w837 -> [w841 _]
                                frame False {
                                n764 = case shown="False" w841 {
                                tunnel: w843 -> [w846 w848]
                                tunnel: w842 -> [w845 w847]
                                frame False {
                                n765 = local write "EMER STOP ACK"(FALSE ("EMER STOP ACK")) -> ()
                                n766 = VISA Write(VISA resource name=w846, write buffer=w845) -> ()  [unwired: 1 in, 3 out]
                                }
                                frame True {
                                n767 = local write "EMER STOP ACK"(FALSE ("EMER STOP ACK")) -> ()
                                n768 = VISA Write(VISA resource name=w848, write buffer=w847) -> ()  [unwired: 1 in, 3 out]
                                }
                                }
                                }
                                frame True {
                                n769 = local write "EMER STOP ACK"(TRUE ("EMER STOP ACK")) -> ()
                                }
                              }
                            }
                            frame #1 {
                              n770 = local read "COM Port"() -> (w851:refnum<visa-resource-name>)
                              n771 = VISA Flush I/O Buffer(VISA resource name=w851) -> ()  [unwired: 1 in, 3 out]
                            }
                          }
                          n772 = local read "EMER STOP ACK"() -> (w834:bool)
                        }
                      }
                      frame #3 {
                        w855 = FALSE ("Read out")
                        n773 = local read "IMAQ USB Session Out"() -> (w857:T2)
                        n774 = local read "Image out"() -> (w856:T1)
                        n775 = local read "IMAQ USB Session Out 2"() -> (w853:T2)
                        n776 = local read "Image"() -> (w852:T1)
                        n777 = call "IMAQ Dispose"("Image"=w852) -> ()  [unwired: 2 in, 4 out]
                        n778 = call "IMAQ Dispose"("Image"=w856) -> ()  [unwired: 2 in, 4 out]
                        n779 = call <vilib>:"IMAQ USB Close.vi"("IMAQ USB Session In"=w857) -> ()  [unwired: 1 in, 10 out]
                        n780 = call <vilib>:"IMAQ USB Close.vi"("IMAQ USB Session In"=w853) -> ()  [unwired: 1 in, 10 out]
                        n781 = local read "COM Port"() -> (w854:refnum<visa-resource-name>)
                        n782 = VISA Close(VISA resource name=w854) -> ()  [unwired: 1 in, 1 out]
                        n783 = local write "Syringe Back"(w855) -> ()
                        n784 = local write "Syringe Ind"(w855) -> ()
                        n785 = local write "Wash"(w855) -> ()
                        n786 = local write "Inj Ind"(w855) -> ()
                        n787 = local write "Injection"(w855) -> ()
                        n788 = local write "Cap Ind"(w855) -> ()
                        n789 = local write "capture"(w855) -> ()
                        n790 = local write "Wash Ind"(w855) -> ()
                      }
                      frame #4 {
                        n791 = invoke on="Image" class="ImageControl" method="Reinit To Default"() -> ()  [unwired: 3 in, 3 out]
                      }
                      frame #5 {
                        n792 = local write "Emergency\nStop"(FALSE ("Stop")) -> ()
                        n793 = disable-structure shown="Disabled" {
                          frame Disabled {
                            n794 = Stop(stop? (T)=TRUE) -> ()
                          }
                          frame Enabled {
                          }
                        }
                      }
                    }
                  }
                }
                "Stop 2" <- "Emergency\nStop"
              }
            }
          }
          n795 = while {
            stop <- FALSE stop-if-true
            n796 = disable-structure shown="Enabled" {
              frame Enabled {
                n797 = disable-structure shown="Disabled" {
                  frame Disabled {
                    n798 = call <vilib>:"IMAQ USB Enumerate Cameras.vi"() -> ("USB Camera Names"=w90:string[])  [unwired: 1 in, 10 out]
                    n799 = Search 1D Array(1D array=w90, element="uEye Capture Device 1\u0000", start index (0)=0) -> (index of element=w93:i32)
                    n800 = Index Array(array=w90, index=w93) -> ()  [unwired: 1 out]
                  }
                  frame Enabled {
                  }
                }
                n801 = call <vilib>:"IMAQ USB Enumerate Cameras.vi"() -> ("USB Camera Names"=w80:string[])  [unwired: 1 in, 10 out]
                "USB Camera Names" <- w80
                n802 = Search 1D Array(1D array=w80, element="uEye Capture Device 1\u0000", start index (0)=0) -> (index of element=w79:i32)
                n803 = Index Array(array=w80, index=w79) -> (element=w89:string)
                "USB Camera" <- w89
                n804 = call <vilib>:"IMAQ USB Init.vi"("USB Camera Name"=w89) -> ("IMAQ USB Session Out"=w87:T2)  [unwired: 2 in, 8 out]
                "IMAQ USB Session Out 2" <- w87
                n805 = call "IMAQ Create"("Image Name"="image") -> ("New Image"=w85:T1)  [unwired: 3 in, 2 out]
                n806 = call <vilib>:"IMAQ USB Grab Setup.vi"("IMAQ USB Session In"=w87) -> ("IMAQ USB Session Out"=w84:T2)  [unwired: 1 in, 9 out]
                n807 = while {
                  tunnel: w85 -> [w100]
                  tunnel: w84 -> [w101]
                  tunnel: [w99] -> w83
                  tunnel: [w97] -> w82
                  stop <- FALSE stop-if-true
                  w96 = T5 0 items=["no dialog", "OK message", "continue or stop message", "OK message + warnings", "continue/stop + warnings"] ("type of dialog (OK msg:1)")
                  (unwired) -1074396024 ("error code (no error:0)")
                  n808 = global read "Image Acq..vi" "Image Acq."() -> (w94:bool)
                  "Image Acq." <- w94
                  n809 = case shown="False" w94 {
                    tunnel: w101 -> [w106 w108]
                    tunnel: w100 -> [w105 w107]
                    tunnel: [w104 w108] -> w99
                    tunnel: [w103 w107] -> w97
                    tunnel: [w102 _] -> w95
                    frame False {
                      n810 = call <vilib>:"IMAQ USB Grab Acquire.vi"("Image in"=w105, "IMAQ USB Session In"=w106) -> ("error out"=w102:errorcluster, "Image out"=w103:T1, "IMAQ USB Session Out"=w104:T2)  [unwired: 1 in, 6 out]
                    }
                    frame True {
                    }
                  }
                  "Image" <- w97
                  n811 = call <vilib>:"Simple Error Handler.vi"("type of dialog (OK msg:1)"=w96, "error in (no error)"=w95) -> ()  [unwired: 8 out]
                }
                "IMAQ USB Session Out" <- w83
                "Image out" <- w82
                n812 = call <vilib>:"IMAQ USB Close.vi"("IMAQ USB Session In"=w83) -> ("error out"=w86:errorcluster)  [unwired: 1 in, 9 out]
                n813 = call "IMAQ Dispose"("Image"=w82) -> ()  [unwired: 2 in, 4 out]
                n814 = call <vilib>:"Simple Error Handler.vi"("error in (no error)"=w86) -> ()  [unwired: 1 in, 8 out]
              }
              frame Disabled {
                n815 = while {
                  tunnel: [w116] -> _
                  tunnel: [w115] -> _
                  stop <- w113 stop-if-true
                  w111 = T5 0 items=["no dialog", "OK message", "continue or stop message", "OK message + warnings", "continue/stop + warnings"] ("type of dialog (OK msg:1)")
                  n816 = global read "Image Acq..vi" "Image Acq."() -> (w114:bool)
                  n817 = call <vilib>:"IMAQ USB Grab Acquire.vi"() -> ("error out"=w110:errorcluster, "Image out"=w115:T1, "IMAQ USB Session Out"=w116:T2)  [unwired: 3 in, 6 out]
                  n818 = Not(x=w114) -> (.not. x?=w113:bool)
                  n819 = call <vilib>:"Simple Error Handler.vi"("error code (no error:0)"=-1074396024, "type of dialog (OK msg:1)"=w111, "error in (no error)"=w110) -> ()  [unwired: 7 out]
                }
                n820 = local read "COM Port"() -> (w109:refnum<visa-resource-name>)
                n821 = VISA Flush I/O Buffer(VISA resource name=w109) -> ()  [unwired: 1 in, 3 out]
              }
            }
          }
        }
      }
    }
  }
  n822 = disable-structure shown="Disabled" {
    frame Disabled {
      (unwired) path "C:/hasan1.jpg" ("File Path")
      (unwired) FALSE ("x = y?")
      (unwired) FALSE ("x = y?")
      w866 = T5 0 items=["no dialog", "OK message", "continue or stop message", "OK message + warnings", "continue/stop + warnings"] ("type of dialog (OK msg:1)")
      w867 = T6 1073684533 items=["Service Request"=1073684491, "Trigger"=3221168138, "Clear"=1073684493, "VXI Signal"=1073684512, "VXI/VME Interrupt"=3221168161, "VXI/VME Sysfail"=1073684509, "VXI/VME Sysreset"=1073684510, "GPIB CIC"=1073684498, "GPIB Talk"=1073684499, "GPIB Listen"=1073684500, "PXI Interrupt"=1073684514, "Serial Break"=1073684515, "Serial TermChar"=1073684516, "Serial CTS"=1073684521, "Serial DSR"=1073684522, "Serial DCD"=1073684524, "Serial RI"=1073684526, "Serial Character"=1073684533, "USB Interrupt"=1073684535, "All Enabled"=1073709055] ("Event Type")
      # "RX Selector\n1 Wash Begin\n2 Wash End"
      n823 = Type Cast() -> ()  [unwired: 1 in, 2 out]
      n824 = local read "COM Port"() -> (w868:refnum<visa-resource-name>)
      n825 = stacked-sequence {
        tunnel: [_ _ w874] -> _
        frame #0 {
          (unwired) i8 66 items=["Syringe"=83, "Temp"=84, "Pump"=80, "Walve "=86, "LED "=76, "JIG "=74, "Wash"=65, "Injection"=66, "Capture"=67, "Readout"=68]  # Commands
          (unwired) i8 48 items=["STOP"=48, "Begin"=49]  # DATAs  Control
          n826 = stacked-sequence {
            frame #0 {
            }
          }
        }
        frame #1 {
          w871 = i8 49 items=["Write Command"=49]  # DATAs Command
          w872 = i8 50  # Data Length
          w873 = i8 72  # Header
          n827 = Compound Arithmetic op=ADD(w873, w872, w871) -> ()  [unwired: 2 in, 1 out]
        }
        frame #2 {
          w882 = i8 50  # Data Length
          w883 = i8 72  # Header
          w881 = i8 49 items=["Write Command"=49]  # DATAs Command
          n828 = Type Cast(x=w883) -> (*(type *) &x=w880:string)  [unwired: 1 out]
          n829 = Type Cast() -> (*(type *) &x=w875:string)  [unwired: 1 in, 1 out]
          n830 = Type Cast(x=w881) -> (*(type *) &x=w877:string)  [unwired: 1 out]
          n831 = Type Cast() -> (*(type *) &x=w876:string)  [unwired: 1 in, 1 out]
          n832 = Type Cast() -> (*(type *) &x=w879:string)  [unwired: 1 in, 1 out]
          n833 = Type Cast(x=w882) -> (*(type *) &x=w878:string)  [unwired: 1 out]
          n834 = Concatenate Strings(w880, w879, w878, w877, w876, w875) -> (w874:string)
        }
      }
      n835 = Equal?() -> ()  [unwired: 2 in, 1 out]
      n836 = local read "COM Port"() -> (w862:refnum<visa-resource-name>)
      n837 = local read "AutoStart"() -> ()  [unwired: 1 in]
      n838 = local read "Inj ACK"() -> ()  [unwired: 1 in]
      n839 = VISA Enable Event(10:w867, 11:w868) -> (3:w870:refnum<visa-resource-name>)  [unwired: 1 in, 2 out]
      n840 = property on="AutoStart" class="Bool (strict)"("Disabled"=u8 2) -> ()  [unwired: 2 in, 2 out]
      n841 = VISA Wait on Event(11:w870) -> (3:→"Read RX":refnum<visa-resource-name>)  [unwired: 1 in, 6 out]
      n842 = VISA Flush I/O Buffer(VISA resource name=w862) -> ()  [unwired: 1 in, 3 out]
      n843 = while {
        stop <- _ stop-if-true
      }
      n844 = local read "Syringe Back"() -> ()  [unwired: 1 in]
      n845 = local read "EMER STOP ACK"() -> ()  [unwired: 1 in]
      n846 = flat-sequence {
        frame #0 {
        }
      }
      n847 = global read "Set_Cancel.vi" "Cancel"() -> ()  [unwired: 1 out]
      n848 = case shown="True" {
        selector: _ -> [_ _]
        frame False {
        }
        frame True {
        }
      }
      n849 = local read "Wash"() -> ()  [unwired: 1 out]
      n850 = call <vilib>:"Simple Error Handler.vi"("error code (no error:0)"=-1073807339, "type of dialog (OK msg:1)"=w866) -> ()  [unwired: 1 in, 7 out]
      n851 = local read "COM Port"() -> (w864:refnum<visa-resource-name>)
      n852 = local read "Autostart Ind"() -> ()  [unwired: 1 in]
      n853 = local read item#-1() -> ()  [unwired: 1 in]
      n854 = VISA Write(VISA resource name=w864) -> ()  [unwired: 2 in, 3 out]
      n855 = Wait Until Next ms Multiple(millisecond multiple=u32 1) -> ()  [unwired: 1 out]
      n856 = local read "Wash ACK"() -> ()  [unwired: 1 out]
      n857 = Wait Until Next ms Multiple(millisecond multiple=u32 100) -> ()  [unwired: 1 out]
    }
    frame Enabled {
    }
  }
  n858 = while {
    i -> [w885]
    stop <- FALSE stop-if-true
    n859 = case shown="True" "Mal Func Stop" {
      selector: "Mal Func Stop" -> [_ w887]
      frame False {
      }
      frame True {
        n860 = stacked-sequence {
          tunnel: w887 -> [_ _]
          frame #0 {
            n861 = local read "Image"() -> (w888:T1)
            n862 = invoke on="Image" class="ImageControl" method="Reinit To Default"() -> ()  [unwired: 3 in, 3 out]
            n863 = call "IMAQ Dispose"("Image"=w888) -> ()  [unwired: 2 in, 4 out]
            n864 = local read "IMAQ USB Session Out 2"() -> (w889:T2)
            n865 = local read "IMAQ USB Session Out"() -> (w891:T2)
            n866 = local read "Image out"() -> (w890:T1)
            n867 = call "IMAQ Dispose"("Image"=w890) -> ()  [unwired: 2 in, 4 out]
            n868 = call <vilib>:"IMAQ USB Close.vi"("IMAQ USB Session In"=w891) -> ()  [unwired: 1 in, 10 out]
            n869 = call <vilib>:"IMAQ USB Close.vi"("IMAQ USB Session In"=w889) -> ()  [unwired: 1 in, 10 out]
          }
          frame #1 {
            n870 = Stop(stop? (T)=TRUE) -> ()
          }
        }
        n871 = global write "malfunc. stop.vi" "Mal func.  Stop"(w887) -> ()
      }
    }
    "Numeric" <- w885
  }
